vi "总磷总氮通讯.vi"() -> ()   [LabVIEW 2016, in "斯坦道氟化物.lvlib"]
uses:
  <vilib>/Plasmionique/MB Master/MB_Master_Serial/MB_Master_Serial.lvclass
  E:/Program Files (x86)/National Instruments/LabVIEW 2016/vi.lib/Plasmionique/MB Master/MB_Master/MB_Master.lvclass
  <vilib>/Plasmionique/MB Master/MB_Master_TCP/MB_Master_TCP.lvclass
  <vilib>/Utility/config.llb/Write Key (Boolean).vi
  <vilib>/Utility/config.llb/Write Key (String).vi
  <vilib>/Plasmionique/MB Master/MB_Master/MB_Master.lvclass
  <vilib>/Utility/config.llb/NI_LVConfig.lvlib
  <vilib>/Plasmionique/MB Master/MB Master.lvlib
  <vilib>/ptbypt/NI_PtbyPt.lvlib
panel:
  out "启用":bool=TRUE
  out "氨氮状态告警区":u16[](array[numeric])
  out "氨氮测量数据区":u16[](array[numeric])
  out "COD测量数据区":u16[](array[numeric])
  out "COD状态告警区":u16[](array[numeric])
  out "总氮测量数据区":u16[](array[numeric])
  out "总氮状态告警区":u16[](array[numeric])
  out "总磷状态告警区":u16[](array[numeric])
  out "总磷测量数据区":u16[](array[numeric])
  out "状态告警区":T1 {"告警代码" items=["无告警", "缺试剂告警", "缺水样告警", "缺蒸馏水告警", "缺标液告警", "仪表漏液告警", "标定异常告警", "超量程告警", "加热异常", "低试剂预警", "超上限告警", "超下限告警", "仪表内部其他异常", "滴定异常告警", "电极异常告警", "量程切换告警", "参数设置告警", "PH电极电位异常", "电导率电极异常", "浊度光度异常", "溶解氧电极异常", "溶解氧光强异常", "温度异常告警", "PH异常告警", "溶解氧异常告警", "电导率异常告警", "浊度异常告警", "叶绿素异常告警", "藻密度异常告警", "蓝绿藻异常告警", "ORP异常告警", "氨氮异常告警", "清洁刷异常告警", "SD卡异常告警", "蓝牙异常告警", "Wifi异常告警", "流程异常告警"]; "故障代码" items=["无故障", "电机故障", "温度故障", "通讯故障", "滴定故障"]}
  out "测量数据区":T2 {"单位" items=["ug/L", "mg/L", "ppm", "mg/m3", "cm", "ppb", "ug/m3", "%", "nmol/mol", "umol/mol", "MPN/L", "MPN/100ml", "ng/m3", "NTU", "无量纲", "ms/cm", "us/cm", "℃", "mV", "万个/L"]}
  out "status":bool
  out "关键参数区":T3
  in  "读关键参数区":bool
  in  "读状态告警区":bool
  in  "读测量数据区":bool
  in  "站号":u16(ring) items=["总磷"=1, "氨氮"=3]
  in  "停止":bool
  in  "启动":bool
  in  "控制命令":u16(ring) items=["启动测量"=1, "标样核查"=2, "零点核查"=3, "跨度核查"=4, "空白测试"=5, "平行样测试"=6, "加标回收"=7, "空白校准"=8, "标样校准"=9, "初始化（清洗）"=10, "停止测试"=11, "仪器重启"=12, "校时"=13, "模式设置"=14, "测量间隔设置"=15]
  in  "控制命令参数":u16[](array[numeric]) format="%04xH"
  in  "VISA Resource":refnum<visa-resource-name>
  in  "启用模块":bool
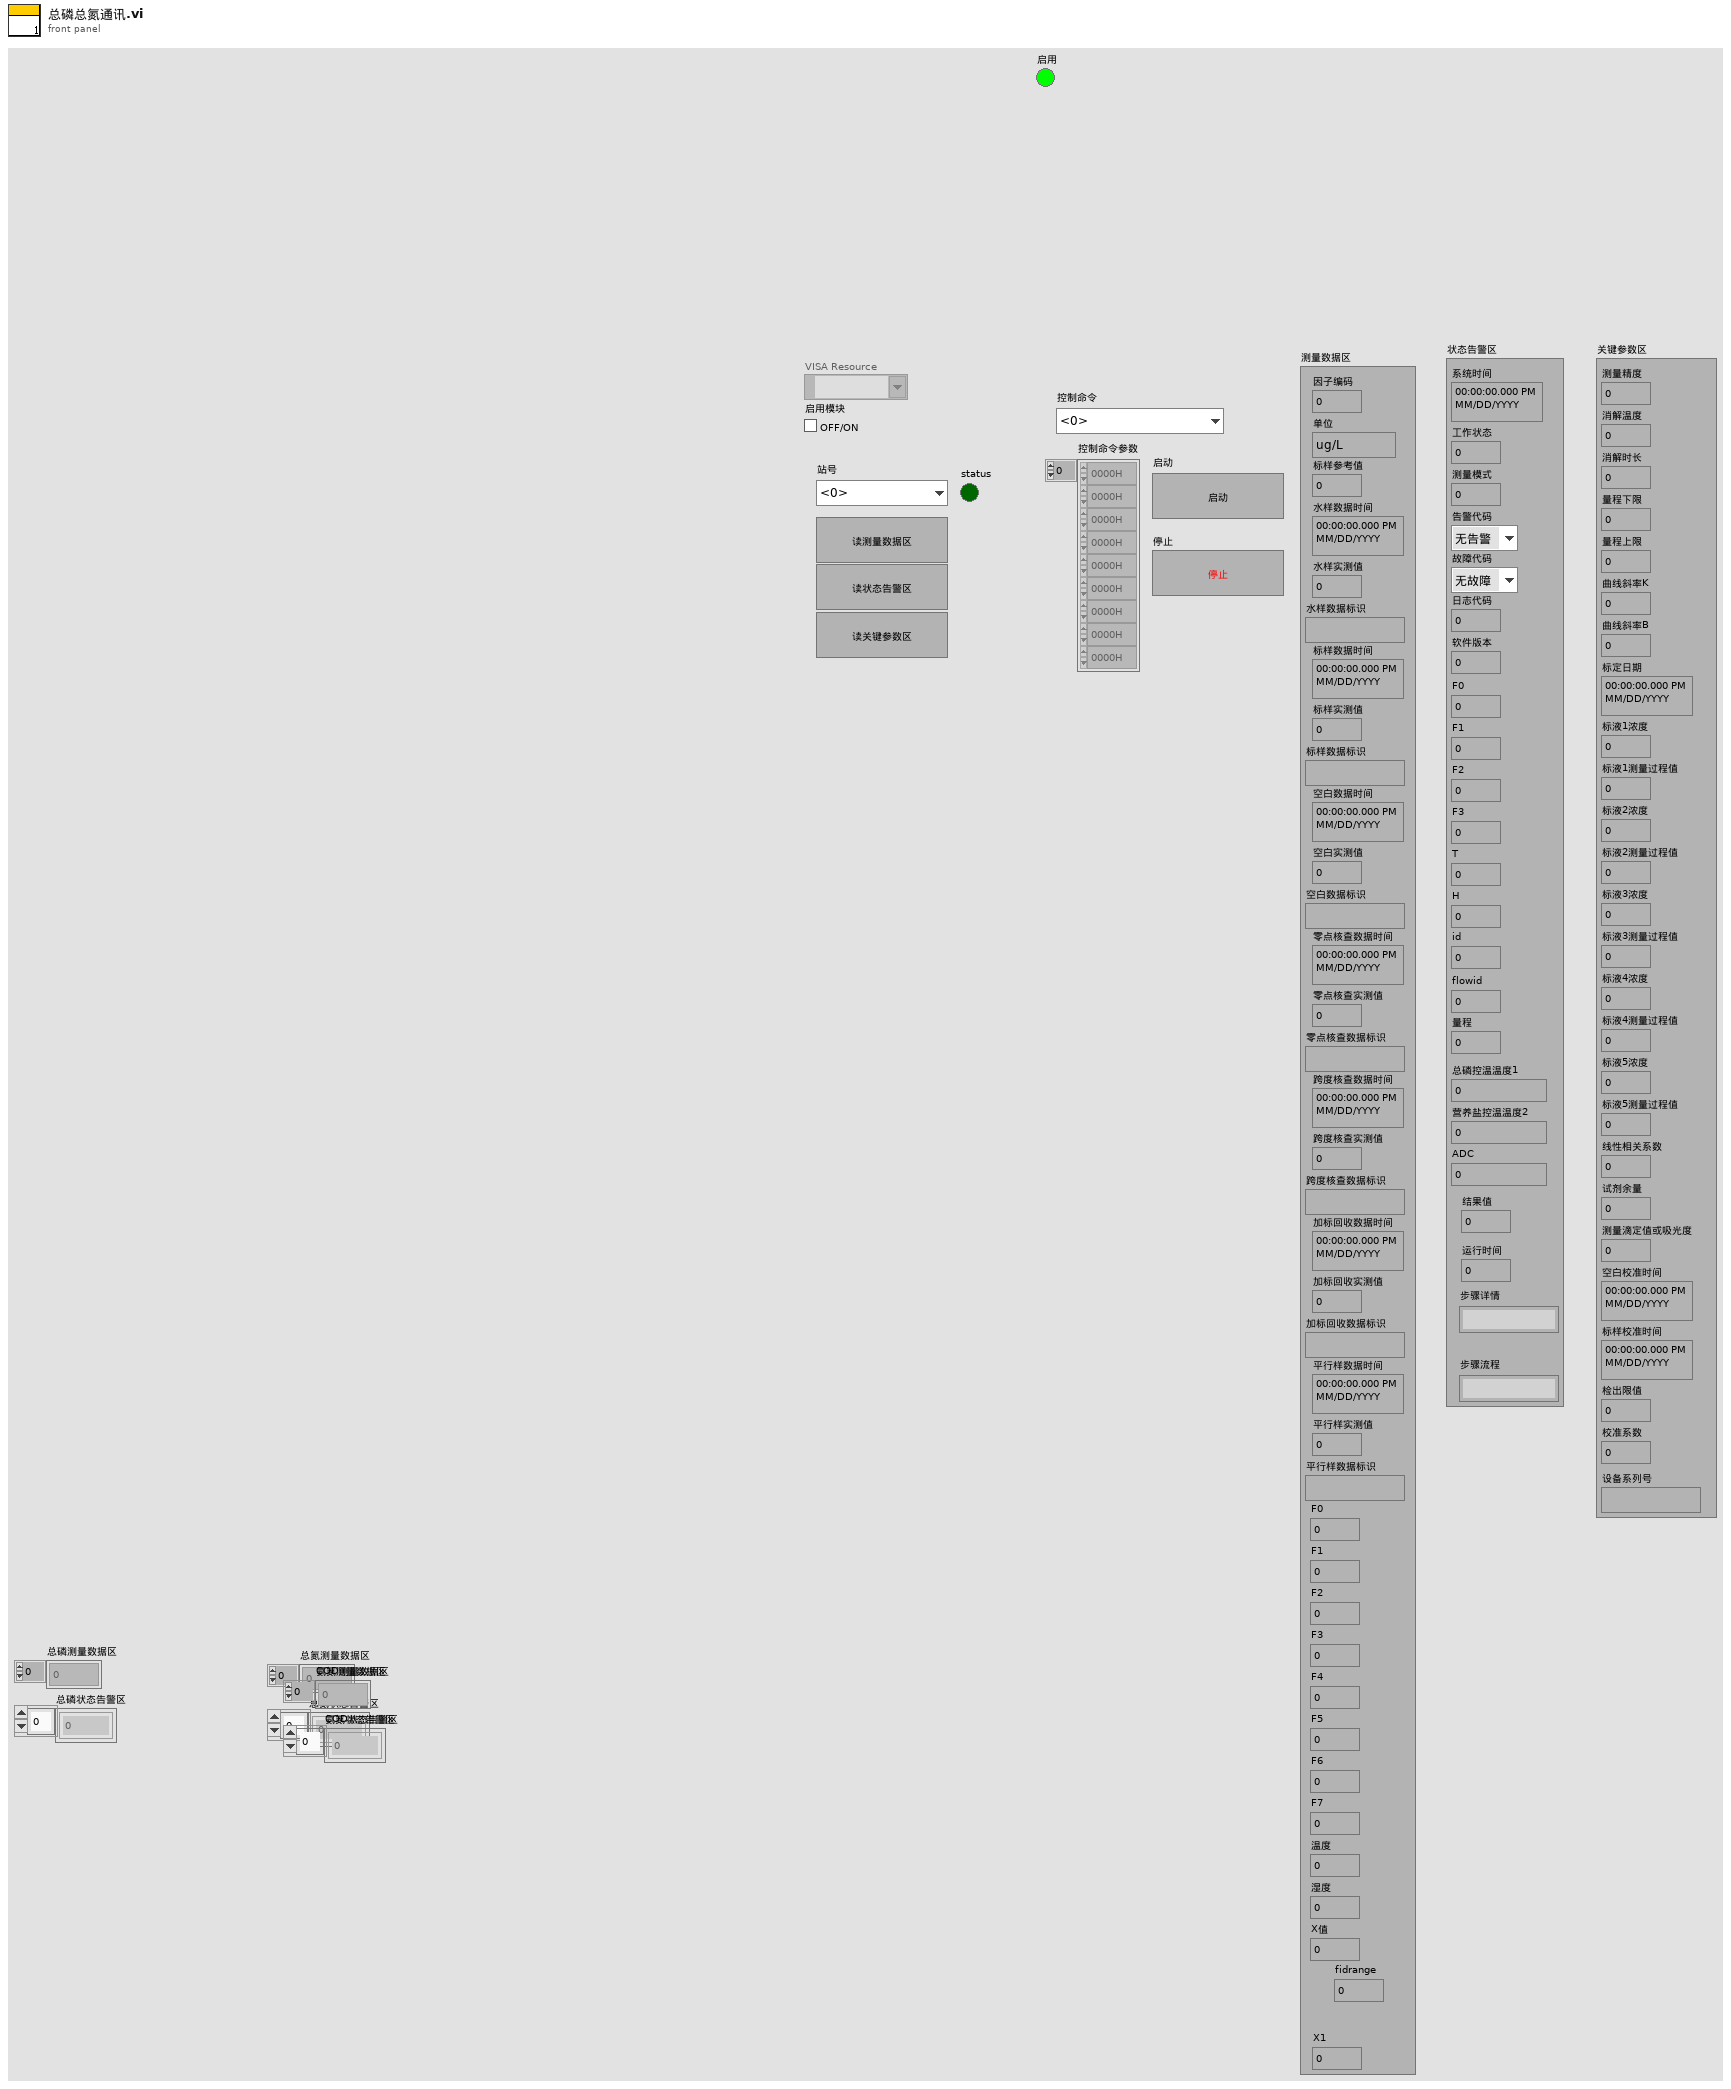
[diagram p1: front panel]
types:
  T1 = cluster{"系统时间":timestamp, "工作状态":u16, "测量模式":u16, "告警代码":u16, "故障代码":u16, "日志代码":u16, "软件版本":u16, "F0":sgl, "F1":sgl, "F2":sgl, "F3":sgl, "T":sgl, "H":sgl, "id":u16, "flowid":u16, "量程":u16, "总磷控温温度1":sgl, "营养盐控温温度2":sgl, "ADC":sgl, "结果值":sgl, "运行时间":u16, "步骤详情":string, "步骤流程":string}
  T2 = cluster{"因子编码":u32, "单位":u16, "标样参考值":sgl, "水样数据时间":timestamp, "水样实测值":sgl, "水样数据标识":string, "标样数据时间":timestamp, "标样实测值":sgl, "标样数据标识":string, "空白数据时间":timestamp, "空白实测值":sgl, "空白数据标识":string, "零点核查数据时间":timestamp, "零点核查实测值":sgl, "零点核查数据标识":string, "跨度核查数据时间":timestamp, "跨度核查实测值":sgl, "跨度核查数据标识":string, "加标回收数据时间":timestamp, "加标回收实测值":sgl, "加标回收数据标识":string, "平行样数据时间":timestamp, "平行样实测值":sgl, "平行样数据标识":string, "F0":sgl, "F1":sgl, "F2":sgl, "F3":sgl, "F4":sgl, "F5":sgl, "F6":sgl, "F7":sgl, "温度":sgl, "湿度":sgl, "X值":sgl, "fidrange":u16, "X1":sgl}
  T3 = cluster{"测量精度":u16, "消解温度":u16, "消解时长":u16, "量程下限":sgl, "量程上限":sgl, "曲线斜率K":sgl, "曲线斜率B":sgl, "标定日期":timestamp, "标液1浓度":sgl, "标液1测量过程值":sgl, "标液2浓度":sgl, "标液2测量过程值":sgl, "标液3浓度":sgl, "标液3测量过程值":sgl, "标液4浓度":sgl, "标液4测量过程值":sgl, "标液5浓度":sgl, "标液5测量过程值":sgl, "线性相关系数":sgl, "试剂余量":u32, "测量滴定值或吸光度":sgl, "空白校准时间":timestamp, "标样校准时间":timestamp, "检出限值":sgl, "校准系数":sgl, "设备系列号":string}
  T4 = cluster{"系统时间":timestamp, "工作状态":u16, "测量模式":enum16{"待机", "连续模式", "周期模式", "定点模式", "受控模式", "手动模式"}, "告警代码":u16, "故障代码":u16, "日志代码":u16, "软件版本":u16, "F0":sgl, "F1":sgl, "F2":sgl, "F3":sgl, "T":sgl, "H":sgl, "id":u16, "flowid":u16, "量程":u16, "总磷控温温度1":sgl, "营养盐控温温度2":sgl, "ADC":sgl}
  T5 = cluster{"因子编码":u32, "单位":u16, "标样参考值":sgl, "水样数据时间":timestamp, "水样实测值":sgl, "水样数据标识":string, "标样数据时间":timestamp, "标样实测值":sgl, "标样数据标识":string, "空白数据时间":timestamp, "空白实测值":sgl, "空白数据标识":string, "零点核查数据时间":timestamp, "零点核查实测值":sgl, "零点核查数据标识":string, "跨度核查数据时间":timestamp, "跨度核查实测值":sgl, "跨度核查数据标识":string, "加标回收数据时间":timestamp, "加标回收实测值":sgl, "加标回收数据标识":string, "平行样数据时间":timestamp, "平行样实测值":sgl, "平行样数据标识":string, "F0":sgl, "F1":sgl, "F2":sgl, "F3":sgl, "F4":sgl, "F5":sgl, "F6":sgl, "F7":sgl, "温度":sgl, "湿度":sgl, "X值":sgl, "fidrange":u16, "X1值":sgl}
  T6 = cluster{"测量精度":u16, "消解温度":u16, "消解时长":u16, "量程下限":sgl, "量程上限":sgl, "曲线斜率K":sgl, "曲线斜率B":sgl, "标定日期":timestamp, "标液1浓度":sgl, "标液1测量过程值":sgl, "标液2浓度":sgl, "标液2测量过程值":sgl, "标液3浓度":sgl, "标液3测量过程值":sgl, "标液4浓度":sgl, "标液4测量过程值":sgl, "标液5浓度":sgl, "标液5测量过程值":sgl, "线性相关系数":sgl, "试剂余量":u32, "测量滴定值或吸光度":sgl, "空白校准时间":timestamp, "标样校准时间":timestamp, "检出限值":sgl, "校准系数":sgl, "设备系列号":string}[]
  T7 = cluster{"系统时间":timestamp, "工作状态":u16, "测量模式":enum16{"待机", "连续模式", "周期模式", "定点模式", "受控模式", "手动模式"}, "告警代码":u16, "故障代码":u16, "日志代码":u16, "软件版本":u16, "F0":sgl, "F1":sgl, "F2":sgl, "F3":sgl, "T":sgl, "H":sgl, "id":u16, "flowid":u16, "量程":u16, "总磷控温温度1":sgl, "营养盐控温温度2":sgl, "ADC":sgl}[]
  T8 = cluster{"因子编码":u32, "单位":u16, "标样参考值":sgl, "水样数据时间":timestamp, "水样实测值":sgl, "水样数据标识":string, "标样数据时间":timestamp, "标样实测值":sgl, "标样数据标识":string, "空白数据时间":timestamp, "空白实测值":sgl, "空白数据标识":string, "零点核查数据时间":timestamp, "零点核查实测值":sgl, "零点核查数据标识":string, "跨度核查数据时间":timestamp, "跨度核查实测值":sgl, "跨度核查数据标识":string, "加标回收数据时间":timestamp, "加标回收实测值":sgl, "加标回收数据标识":string, "平行样数据时间":timestamp, "平行样实测值":sgl, "平行样数据标识":string, "F0":sgl, "F1":sgl, "F2":sgl, "F3":sgl, "F4":sgl, "F5":sgl, "F6":sgl, "F7":sgl, "温度":sgl, "湿度":sgl, "X值":sgl, "fidrange":u16, "X1值":sgl}[]
  T9 = typedef "CODCr交互.ctl" = cluster{"状态告警区":cluster{"系统时间":timestamp, "工作状态":u16, "测量模式":enum16{"待机", "连续模式", "周期模式", "定点模式", "受控模式", "手动模式"}, "告警代码":u16, "故障代码":u16, "日志代码":u16, "软件版本":u16, "F0":sgl, "F1":sgl, "F2":sgl, "F3":sgl, "T":sgl, "H":sgl, "id":u16, "flowid":u16, "量程":u16, "总磷控温温度1":sgl, "营养盐控温温度2":sgl, "ADC":sgl}, "平台试剂余量百分比":sgl, "关键参数":cluster{"测量量程":dbl, "测量精度":dbl, "测量间隔":dbl, "消解温度":dbl, "消解时长":dbl, "空白校准时间":timestamp, "曲线截距":dbl, "曲线斜率":dbl, "测量检出限":dbl, "测量信号值":dbl, "线性相关系数":dbl, "二次多项式系数":dbl, "标样校准时间":timestamp, "稀释倍数":dbl, "三项式系数":dbl, "空白标定系数":dbl, "量程系数":dbl, "F0/ORPA":dbl, "F1/ORPB":dbl, "F2/ORPK":dbl, "F3":dbl, "F4":dbl, "F5":dbl, "F6":dbl, "F7":dbl, "X0/滴定数":dbl, "量程":dbl}, "关键参数改变":bool, "校准信息":cluster{"低标液1浓度":dbl, "低标液1信号值":dbl, "低标液1启用":u16, "低标液2浓度":dbl, "低标液2信号值":dbl, "低标液2启用":u16, "低标液3浓度":dbl, "低标液3信号值":dbl, "低标液3启用":u16, "低标液4浓度":dbl, "低标液4信号值":dbl, "低标液4启用":u16, "低标液5浓度":dbl, "低标液5信号值":dbl, "低标液5启用":u16, "高标液1浓度":dbl, "高标液1信号值":dbl, "高标液1启用":u16, "高标液2浓度":dbl, "高标液2信号值":dbl, "高标液2启用":u16, "高标液3浓度":dbl, "高标液3信号值":dbl, "高标液3启用":u16, "高标液4浓度":dbl, "高标液4信号值":dbl, "高标液4启用":u16, "高标液5浓度":dbl, "高标液5信号值":dbl, "高标液5启用":u16, "低斜率":dbl, "低截距":dbl, "低二次多项式系数":dbl, "低线性相关系数":dbl, "高斜率":dbl, "高截距":dbl, "高二次多项式系数":dbl, "高线性相关系数":dbl}, "校准信息改变":bool, "固件版本号":string}
  T10 = typedef "总磷交互.ctl" = cluster{"状态告警区":cluster{"系统时间":timestamp, "工作状态":u16, "测量模式":enum16{"待机", "连续模式", "周期模式", "定点模式", "受控模式", "手动模式"}, "告警代码":u16, "故障代码":u16, "日志代码":u16, "软件版本":u16, "F0":sgl, "F1":sgl, "F2":sgl, "F3":sgl, "T":sgl, "H":sgl, "id":u16, "flowid":u16, "量程":u16, "总磷控温温度1":sgl, "营养盐控温温度2":sgl, "ADC":sgl}, "平台试剂余量百分比":sgl, "关键参数":cluster{"测量量程":dbl, "测量精度":dbl, "测量间隔":dbl, "消解温度":dbl, "消解时长":dbl, "空白校准时间":timestamp, "曲线截距":dbl, "曲线斜率":dbl, "测量检出限":dbl, "测量信号值":dbl, "线性相关系数":dbl, "二次多项式系数":dbl, "标样校准时间":timestamp, "稀释倍数":dbl, "三项式系数":dbl, "空白标定系数":dbl, "量程系数":dbl, "F0/ORPA":dbl, "F1/ORPB":dbl, "F2/ORPK":dbl, "F3":dbl, "F4":dbl, "F5":dbl, "F6":dbl, "F7":dbl, "X0/滴定数":dbl, "量程":dbl}, "关键参数改变":bool, "校准信息":cluster{"低标液1浓度":dbl, "低标液1信号值":dbl, "低标液1启用":u16, "低标液2浓度":dbl, "低标液2信号值":dbl, "低标液2启用":u16, "低标液3浓度":dbl, "低标液3信号值":dbl, "低标液3启用":u16, "低标液4浓度":dbl, "低标液4信号值":dbl, "低标液4启用":u16, "低标液5浓度":dbl, "低标液5信号值":dbl, "低标液5启用":u16, "高标液1浓度":dbl, "高标液1信号值":dbl, "高标液1启用":u16, "高标液2浓度":dbl, "高标液2信号值":dbl, "高标液2启用":u16, "高标液3浓度":dbl, "高标液3信号值":dbl, "高标液3启用":u16, "高标液4浓度":dbl, "高标液4信号值":dbl, "高标液4启用":u16, "高标液5浓度":dbl, "高标液5信号值":dbl, "高标液5启用":u16, "低斜率":dbl, "低截距":dbl, "低二次多项式系数":dbl, "低线性相关系数":dbl, "高斜率":dbl, "高截距":dbl, "高二次多项式系数":dbl, "高线性相关系数":dbl}, "校准信息改变":bool, "固件版本号":string}
  T11 = typedef "总氮交互.ctl" = cluster{"状态告警区":cluster{"系统时间":timestamp, "工作状态":u16, "测量模式":enum16{"待机", "连续模式", "周期模式", "定点模式", "受控模式", "手动模式"}, "告警代码":u16, "故障代码":u16, "日志代码":u16, "软件版本":u16, "F0":sgl, "F1":sgl, "F2":sgl, "F3":sgl, "T":sgl, "H":sgl, "id":u16, "flowid":u16, "量程":u16, "总磷控温温度1":sgl, "营养盐控温温度2":sgl, "ADC":sgl}, "平台试剂余量百分比":sgl, "关键参数":cluster{"测量量程":dbl, "测量精度":dbl, "测量间隔":dbl, "消解温度":dbl, "消解时长":dbl, "空白校准时间":timestamp, "曲线截距":dbl, "曲线斜率":dbl, "测量检出限":dbl, "测量信号值":dbl, "线性相关系数":dbl, "二次多项式系数":dbl, "标样校准时间":timestamp, "稀释倍数":dbl, "三项式系数":dbl, "空白标定系数":dbl, "量程系数":dbl, "F0/ORPA":dbl, "F1/ORPB":dbl, "F2/ORPK":dbl, "F3":dbl, "F4":dbl, "F5":dbl, "F6":dbl, "F7":dbl, "X0/滴定数":dbl, "量程":dbl}, "关键参数改变":bool, "校准信息":cluster{"低标液1浓度":dbl, "低标液1信号值":dbl, "低标液1启用":u16, "低标液2浓度":dbl, "低标液2信号值":dbl, "低标液2启用":u16, "低标液3浓度":dbl, "低标液3信号值":dbl, "低标液3启用":u16, "低标液4浓度":dbl, "低标液4信号值":dbl, "低标液4启用":u16, "低标液5浓度":dbl, "低标液5信号值":dbl, "低标液5启用":u16, "高标液1浓度":dbl, "高标液1信号值":dbl, "高标液1启用":u16, "高标液2浓度":dbl, "高标液2信号值":dbl, "高标液2启用":u16, "高标液3浓度":dbl, "高标液3信号值":dbl, "高标液3启用":u16, "高标液4浓度":dbl, "高标液4信号值":dbl, "高标液4启用":u16, "高标液5浓度":dbl, "高标液5信号值":dbl, "高标液5启用":u16, "低斜率":dbl, "低截距":dbl, "低二次多项式系数":dbl, "低线性相关系数":dbl, "高斜率":dbl, "高截距":dbl, "高二次多项式系数":dbl, "高线性相关系数":dbl}, "校准信息改变":bool, "固件版本号":string}
  T12 = typedef "氨氮交互.ctl" = cluster{"状态告警区":cluster{"系统时间":timestamp, "工作状态":u16, "测量模式":enum16{"待机", "连续模式", "周期模式", "定点模式", "受控模式", "手动模式"}, "告警代码":u16, "故障代码":u16, "日志代码":u16, "软件版本":u16, "F0":sgl, "F1":sgl, "F2":sgl, "F3":sgl, "T":sgl, "H":sgl, "id":u16, "flowid":u16, "量程":u16, "总磷控温温度1":sgl, "营养盐控温温度2":sgl, "ADC":sgl}, "平台试剂余量百分比":sgl, "关键参数":cluster{"测量量程":dbl, "测量精度":dbl, "测量间隔":dbl, "消解温度":dbl, "消解时长":dbl, "空白校准时间":timestamp, "曲线截距":dbl, "曲线斜率":dbl, "测量检出限":dbl, "测量信号值":dbl, "线性相关系数":dbl, "二次多项式系数":dbl, "标样校准时间":timestamp, "稀释倍数":dbl, "三项式系数":dbl, "空白标定系数":dbl, "量程系数":dbl, "F0/ORPA":dbl, "F1/ORPB":dbl, "F2/ORPK":dbl, "F3":dbl, "F4":dbl, "F5":dbl, "F6":dbl, "F7":dbl, "X0/滴定数":dbl, "量程":dbl}, "关键参数改变":bool, "校准信息":cluster{"低标液1浓度":dbl, "低标液1信号值":dbl, "低标液1启用":u16, "低标液2浓度":dbl, "低标液2信号值":dbl, "低标液2启用":u16, "低标液3浓度":dbl, "低标液3信号值":dbl, "低标液3启用":u16, "低标液4浓度":dbl, "低标液4信号值":dbl, "低标液4启用":u16, "低标液5浓度":dbl, "低标液5信号值":dbl, "低标液5启用":u16, "高标液1浓度":dbl, "高标液1信号值":dbl, "高标液1启用":u16, "高标液2浓度":dbl, "高标液2信号值":dbl, "高标液2启用":u16, "高标液3浓度":dbl, "高标液3信号值":dbl, "高标液3启用":u16, "高标液4浓度":dbl, "高标液4信号值":dbl, "高标液4启用":u16, "高标液5浓度":dbl, "高标液5信号值":dbl, "高标液5启用":u16, "低斜率":dbl, "低截距":dbl, "低二次多项式系数":dbl, "低线性相关系数":dbl, "高斜率":dbl, "高截距":dbl, "高二次多项式系数":dbl, "高线性相关系数":dbl}, "校准信息改变":bool, "固件版本号":string}
  T13 = typedef "操作日志字段定义.ctl" = cluster{"时间":timestamp, "参数":string, "日志信息":string, "流程参数":string}
  T14 = typedef "NI_LVConfig.lvlib/Config Data RefNum.ctl" = refnum<k1>
  T15 = enum8{"Enabled", "Disabled", "Disabled and Grayed Out"}
  T16 = cluster{"baud rate (bps)":u32, "stop bits":u16, "parity":u16, "flow control":u16, "timeout":u32, "retries":i32}
  T17 = typedef "工况数据.ctl" = cluster{"time":string, "data":cluster{"ups":cluster{"ups":cluster{"input_voltage":ext, "input_frequency":ext, "output_voltage":ext, "output_current":ext, "output_frequency":ext, "output_active_power":ext, "output_apparent_power":ext, "load_rate":ext, "cabinet_temperature":ext, "battery_voltage":ext, "remaining_battery_capacity":ext, "power_on_status":string, "power_supply_mode":string, "fault":bool, "battery_low_voltage":bool, "mains_supply_abnormality":bool}, "启用":bool}, "air_conditioner":cluster{"air_conditioner":cluster{"cabinet_temperature":ext, "air_supply_temperature":ext, "voltage":ext, "current":ext, "compressor_status":string, "Internal_fan_status":string, "external_fan_status":string, "heating_state":string, "refrigeration_state":bool, "high_temperature_alarm":bool, "low_temperature_alarm":bool, "heater_fault":bool, "temperature_sensor_fault":bool, "high_voltage_alarm":bool, "low_voltage_alarm":bool, "refrigeration_start_point":ext, "refrigeration_sensitive_point":ext, "heating_start_point":ext, "heating_sensitive_point":ext, "high_temperature_alarm_point":ext, "low_temperature_alarm_point":ext}, "启用":bool}, "smoke_sensor":cluster{"smoke_sensor":cluster{"trigger_alarm":bool}, "启用":bool}, "water_immersion_sensor":cluster{"water_immersion_sensor":cluster{"trigger_alarm":bool}, "启用":bool}, "temperature_and_humidity_sensor":cluster{"temperature_and_humidity_sensor":cluster{"current_temperature":ext, "current_humidity":ext, "room_temperature_alarm":bool, "humidity_alarm":bool}, "启用":bool}, "gps":cluster{"gps":cluster{"current_longitude":ext, "current_latitude":ext, "launch_longitude":ext, "launch_latitude":ext, "shift_alarm":bool}, "启用":bool}, "solar_controller":cluster{"solar_controller":cluster{"array_voltage":ext, "array_current":ext, "generating_power":ext, "battery_voltage":dbl, "battery_current":ext, "ceiling_voltage":ext, "minimum_voltage":ext, "battery_temperature":ext, "remaining_battery_capacity":ext, "load_voltage":ext, "load_current":ext, "load_power":ext, "equipment_temperature":ext, "accumulated_electricity_consumption_of_the_day":ext, "accumulated_electricity_consumption_of_the_current_month":ext, "accumulated_electricity_consumption_in_the_current_year":ext, "total_accumulated_power_consumption":ext, "accumulated_charging_capacity_of_the_day":ext, "accumulated_charging_amount_of_the_current_month":ext, "accumulated_charging_capacity_of_the_current_year":ext, "total_cumulative_charge":ext}, "启用":bool}, "solar_controller_2":cluster{"solar_controller_2":cluster{"array_voltage":ext, "array_current":ext, "generating_power":ext, "battery_voltage":dbl, "battery_current":ext, "ceiling_voltage":ext, "minimum_voltage":ext, "battery_temperature":ext, "remaining_battery_capacity":ext, "load_voltage":ext, "load_current":ext, "load_power":ext, "equipment_temperature":ext, "accumulated_electricity_consumption_of_the_day":ext, "accumulated_electricity_consumption_of_the_current_month":ext, "accumulated_electricity_consumption_in_the_current_year":ext, "total_accumulated_power_consumption":ext, "accumulated_charging_capacity_of_the_day":ext, "accumulated_charging_amount_of_the_current_month":ext, "accumulated_charging_capacity_of_the_current_year":ext, "total_cumulative_charge":ext}, "启用":bool}, "NH3":cluster{"NH3":cluster{"F0":ext, "F1":ext, "syringe_temperature":ext, "alarm_step":dbl, "X0":ext}, "启用":bool}, "TP":cluster{"TP":cluster{"F0":ext, "F1":ext, "F2":ext, "F3":ext, "digestion_temperature":ext, "constant_temperature":ext, "syringe_temperature":ext, "alarm_step":dbl, "X0":ext}, "启用":bool}, "TN":cluster{"TN":cluster{"F0":ext, "F1":ext, "F2":ext, "F3":ext, "F4":ext, "F5":ext, "F6":ext, "F7":ext, "digestion_temperature":ext, "constant_temperature":ext, "syringe_temperature":ext, "alarm_step":dbl, "X0":ext}, "启用":bool}, "CODMn":cluster{"CODMn":cluster{"temperature_curve":ext[], "titration_curve":ext[], "F0":ext, "F1":ext, "F2":ext, "F3":ext, "F4":ext, "F5":ext, "A":ext, "B":ext, "K":ext}, "启用":bool}, "CODCr":cluster{"CODCr":cluster{"temperature_curve":ext[], "F0":ext, "F1":ext, "reagent_sensor":ext}, "启用":bool}}}
  T18 = cluster{"系统时间":timestamp, "工作状态":u16, "测量模式":enum16{"待机", "连续模式", "周期模式", "定点模式", "受控模式", "手动模式"}, "告警代码":u16, "故障代码":u16, "日志代码":u16, "软件版本":u16, "F0":sgl, "F1":sgl, "F2":sgl, "F3":sgl, "T":sgl, "H":sgl, "id":u16, "flowid":u16, "量程":u16, "总磷控温温度1":sgl, "营养盐控温温度2":sgl, "ADC":sgl, "结果值":sgl, "运行时间":u16, "步骤详情":string, "步骤流程":string}
  T19 = typedef "斯坦道氟化物.lvlib/关键参数.ctl" = cluster{"测量量程":sgl, "测量检出限":sgl, "测量精度":sgl, "测量间隔":sgl, "消解温度":sgl, "消解时长":sgl, "三项式系数":sgl, "二次多项式系数":sgl, "曲线斜率":sgl, "曲线截距":sgl, "线性相关系数":sgl, "空白校准时间":timestamp, "标样校准时间":timestamp, "测量信号值":sgl, "稀释倍数":sgl, "空白标定系数":sgl, "量程系数":sgl}
  T20 = cluster{"测量量程":dbl, "测量精度":dbl, "测量间隔":dbl, "消解温度":dbl, "消解时长":dbl, "空白校准时间":timestamp, "曲线截距":dbl, "曲线斜率":dbl, "测量检出限":dbl, "测量信号值":dbl, "线性相关系数":dbl, "二次多项式系数":dbl, "标样校准时间":timestamp, "稀释倍数":dbl, "三项式系数":dbl, "空白标定系数":dbl, "量程系数":dbl, "F0/ORPA":dbl, "F1/ORPB":dbl, "F2/ORPK":dbl, "F3":dbl, "F4":dbl, "F5":dbl, "F6":dbl, "F7":dbl, "X0/滴定数":dbl, "量程":dbl}
  T21 = cluster{"低标液1浓度":dbl, "低标液1信号值":dbl, "低标液1启用":u16, "低标液2浓度":dbl, "低标液2信号值":dbl, "低标液2启用":u16, "低标液3浓度":dbl, "低标液3信号值":dbl, "低标液3启用":u16, "低标液4浓度":dbl, "低标液4信号值":dbl, "低标液4启用":u16, "低标液5浓度":dbl, "低标液5信号值":dbl, "低标液5启用":u16, "高标液1浓度":dbl, "高标液1信号值":dbl, "高标液1启用":u16, "高标液2浓度":dbl, "高标液2信号值":dbl, "高标液2启用":u16, "高标液3浓度":dbl, "高标液3信号值":dbl, "高标液3启用":u16, "高标液4浓度":dbl, "高标液4信号值":dbl, "高标液4启用":u16, "高标液5浓度":dbl, "高标液5信号值":dbl, "高标液5启用":u16, "低斜率":dbl, "低截距":dbl, "低二次多项式系数":dbl, "低线性相关系数":dbl, "高斜率":dbl, "高截距":dbl, "高二次多项式系数":dbl, "高线性相关系数":dbl}
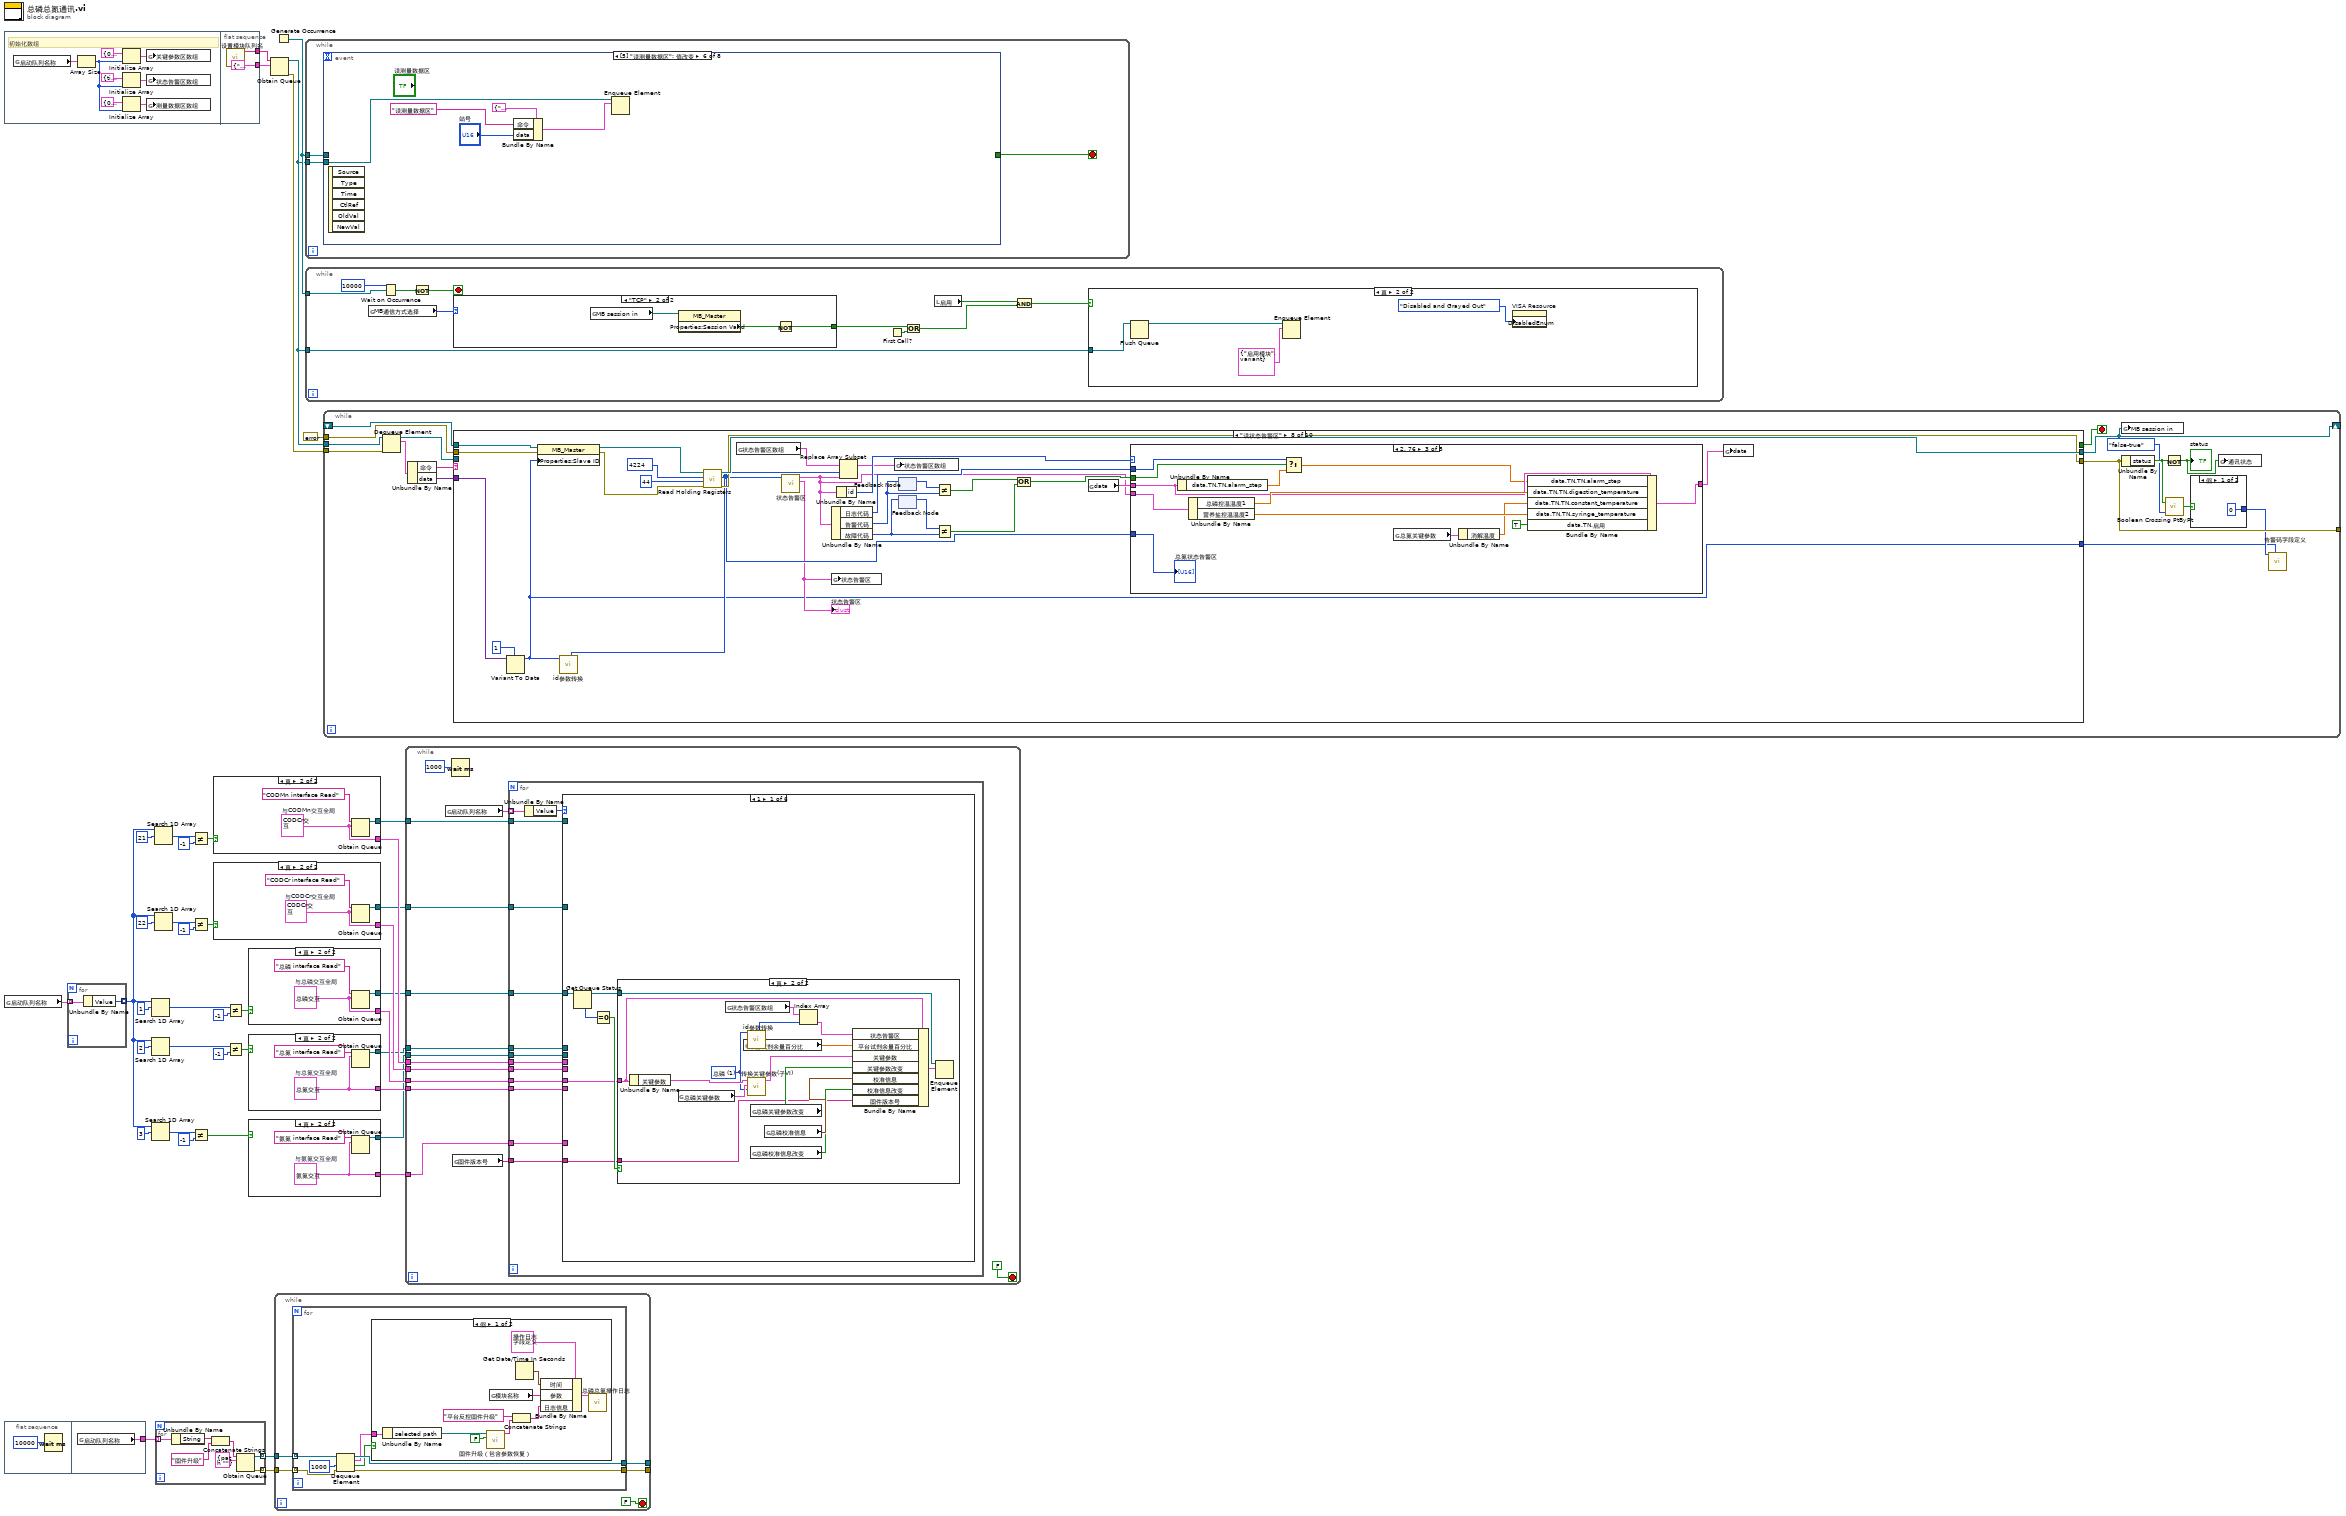
[diagram p0: block diagram]
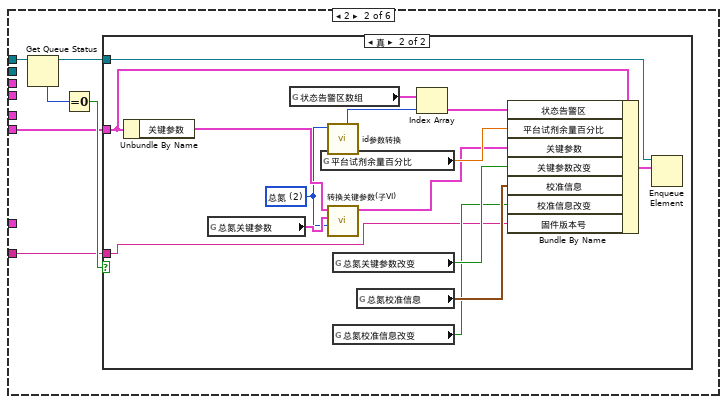
[diagram p9: hidden frame]
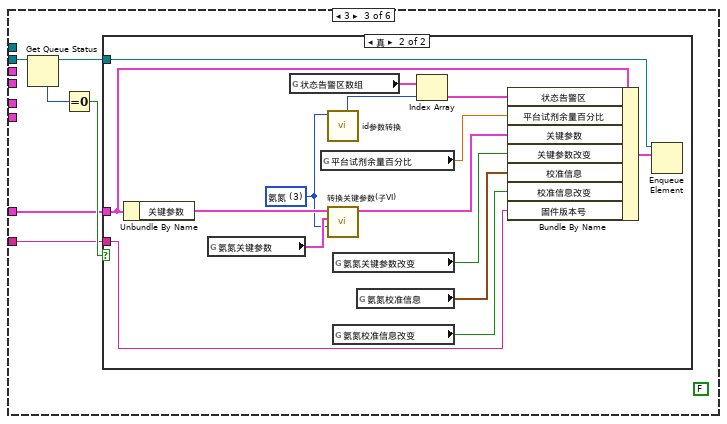
[diagram p11: hidden frame]
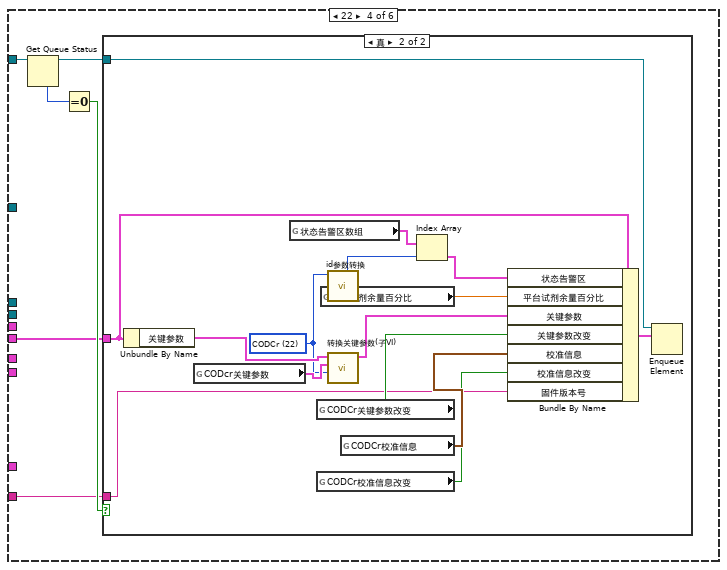
[diagram p13: hidden frame]
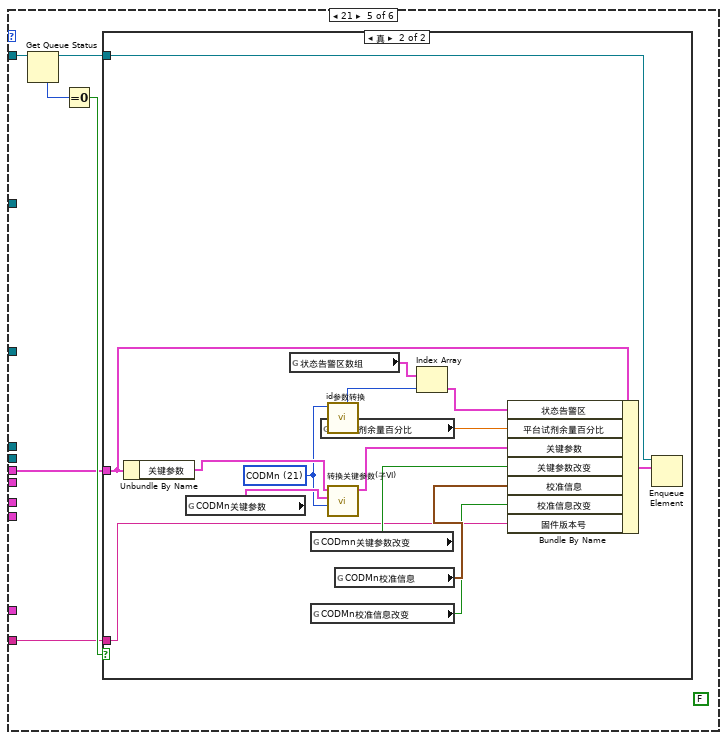
[diagram p15: hidden frame]
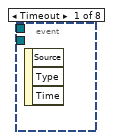
[diagram p20: hidden frame]
diagram:
  n1 = flat-sequence {
    tunnel: [cluster{"命令":string, "data":variant} {"命令"="", "data"=variant}] -> w41
    tunnel: [w50] -> w36
    frame #0 {
      # "初始化数组"
      n2 = global read "model config var.vi" "启动队列名称"() -> (w43:cluster{"String":string, "Value":u16}[])
      n3 = Array Size(array=w43) -> (size(s)=w42:i32)
      n4 = Initialize Array(T3 {"测量精度"=0, "消解温度"=0, "消解时长"=0, "量程下限"=0.0, "量程上限"=0.0, "曲线斜率K"=0.0, "曲线斜率B"=0.0, "标定日期"=timestamp(0 s since 1904-01-01), "标液1浓度"=0.0, "标液1测量过程值"=0.0, "标液2浓度"=0.0, "标液2测量过程值"=0.0, "标液3浓度"=0.0, "标液3测量过程值"=0.0, "标液4浓度"=0.0, "标液4测量过程值"=0.0, "标液5浓度"=0.0, "标液5测量过程值"=0.0, "线性相关系数"=0.0, "试剂余量"=0, "测量滴定值或吸光度"=0.0, "空白校准时间"=timestamp(0 s since 1904-01-01), "标样校准时间"=timestamp(0 s since 1904-01-01), "检出限值"=0.0, "校准系数"=0.0, "设备系列号"=""} ("关键参数区"), w42) -> (w47:T6)
      n5 = Initialize Array(T4 {"系统时间"=timestamp(0 s since 1904-01-01), "工作状态"=0, "测量模式"=enum."待机", "告警代码"=0, "故障代码"=0, "日志代码"=0, "软件版本"=0, "F0"=0.0, "F1"=0.0, "F2"=0.0, "F3"=0.0, "T"=0.0, "H"=0.0, "id"=0, "flowid"=0, "量程"=0, "总磷控温温度1"=0.0, "营养盐控温温度2"=0.0, "ADC"=0.0} ("状态告警区"), w42) -> (w46:T7)
      n6 = Initialize Array(T5 {"因子编码"=0, "单位"=0, "标样参考值"=0.0, "水样数据时间"=timestamp(0 s since 1904-01-01), "水样实测值"=0.0, "水样数据标识"="", "标样数据时间"=timestamp(0 s since 1904-01-01), "标样实测值"=0.0, "标样数据标识"="", "空白数据时间"=timestamp(0 s since 1904-01-01), "空白实测值"=0.0, "空白数据标识"="", "零点核查数据时间"=timestamp(0 s since 1904-01-01), "零点核查实测值"=0.0, "零点核查数据标识"="", "跨度核查数据时间"=timestamp(0 s since 1904-01-01), "跨度核查实测值"=0.0, "跨度核查数据标识"="", "加标回收数据时间"=timestamp(0 s since 1904-01-01), "加标回收实测值"=0.0, "加标回收数据标识"="", "平行样数据时间"=timestamp(0 s since 1904-01-01), "平行样实测值"=0.0, "平行样数据标识"="", "F0"=0.0, "F1"=0.0, "F2"=0.0, "F3"=0.0, "F4"=0.0, "F5"=0.0, "F6"=0.0, "F7"=0.0, "温度"=0.0, "湿度"=0.0, "X值"=0.0, "fidrange"=0, "X1值"=0.0} ("测量数据区"), w42) -> (w49:T8)
      n7 = global write "VAR总磷总氮全局变量.vi" "关键参数区数组"(w47) -> ()
      n8 = global write "VAR总磷总氮全局变量.vi" "状态告警区数组"(w46) -> ()
      n9 = global write "VAR总磷总氮全局变量.vi" "测量数据区数组"(w49) -> ()
    }
    frame #1 {
      n10 = call "设置模块队列名.vi"() -> ("Msg"=w50:string)  [unwired: 5 in]
    }
  }
  n11 = global read "model config var.vi" "启动队列名称"() -> (w25:cluster{"String":string, "Value":u16}[])
  n12 = flat-sequence {
    tunnel: [w53] -> w3
    frame #0 {
      n13 = Wait (ms)(milliseconds to wait=u32 10000 ("等待时间（毫秒）")) -> ()  [unwired: 1 out]
    }
    frame #1 {
      n14 = global read "model config var.vi" "启动队列名称"() -> (w53:cluster{"String":string, "Value":u16}[])
    }
  }
  n15 = for {
    tunnel: w25 -> [w55] mode=indexing
    tunnel: [w54] -> w5 mode=indexing
    n16 = Unbundle By Name(w55) -> ("Value"=w54:u16)
  }
  n17 = Search 1D Array(1D array=w5, element=u16 1 ("元素")) -> (index of element=w15:i32)  [unwired: 1 in]
  n18 = Search 1D Array(1D array=w5, element=u16 2 ("元素")) -> (index of element=w11:i32)  [unwired: 1 in]
  n19 = Search 1D Array(1D array=w5, element=u16 3 ("元素")) -> (index of element=w7:i32)  [unwired: 1 in]
  n20 = Search 1D Array(1D array=w5, element=u16 21 ("元素")) -> (index of element=w23:i32)  [unwired: 1 in]
  n21 = Search 1D Array(1D array=w5, element=u16 22 ("元素")) -> (index of element=w19:i32)  [unwired: 1 in]
  n22 = for {
    tunnel: w3 -> [w62] mode=indexing
    tunnel: [w57] -> w2 mode=indexing
    tunnel: [w56] -> w1 mode=indexing
    n23 = Unbundle By Name(w62) -> ("String"=w58:string)
    n24 = Concatenate Strings(w58, "固件升级" ("字符串")) -> (w60:string)
    n25 = Obtain Queue(name (unnamed)=w60, element data type=cluster{"selected path":path} {"selected path"=path ""}) -> (queue out=w57:refnum<queue>, error out=w56:errorcluster)  [unwired: 3 in, 1 out]
  }
  n26 = Not Equal?(x=w23, y=-1) -> (x != y?=w21:bool)
  n27 = Not Equal?(x=w19, y=-1) -> (x != y?=w17:bool)
  n28 = Not Equal?(x=w7, y=-1) -> (x != y?=w4:bool)
  n29 = case shown="真" w21 {
    tunnel: [_ w64] -> w35
    tunnel: [_ w63] -> w34
    frame False {
    }
    frame True {
      w63 = T9 {"状态告警区"={"系统时间"=timestamp(0 s since 1904-01-01), "工作状态"=0, "测量模式"=enum."待机", "告警代码"=0, "故障代码"=0, "日志代码"=0, "软件版本"=0, "F0"=0.0, "F1"=0.0, "F2"=0.0, "F3"=0.0, "T"=0.0, "H"=0.0, "id"=0, "flowid"=0, "量程"=0, "总磷控温温度1"=0.0, "营养盐控温温度2"=0.0, "ADC"=0.0}, "平台试剂余量百分比"=0.0, "关键参数"={"测量量程"=0.0, "测量精度"=0.0, "测量间隔"=0.0, "消解温度"=0.0, "消解时长"=0.0, "空白校准时间"=timestamp(0 s since 1904-01-01), "曲线截距"=0.0, "曲线斜率"=0.0, "测量检出限"=0.0, "测量信号值"=0.0, "线性相关系数"=0.0, "二次多项式系数"=0.0, "标样校准时间"=timestamp(0 s since 1904-01-01), "稀释倍数"=0.0, "三项式系数"=0.0, "空白标定系数"=0.0, "量程系数"=0.0, "F0/ORPA"=0.0, "F1/ORPB"=0.0, "F2/ORPK"=0.0, "F3"=0.0, "F4"=0.0, "F5"=0.0, "F6"=0.0, "F7"=0.0, "X0/滴定数"=0.0, "量程"=0.0}, "关键参数改变"=FALSE, "校准信息"={"低标液1浓度"=0.0, "低标液1信号值"=0.0, "低标液1启用"=0, "低标液2浓度"=0.0, "低标液2信号值"=0.0, "低标液2启用"=0, "低标液3浓度"=0.0, "低标液3信号值"=0.0, "低标液3启用"=0, "低标液4浓度"=0.0, "低标液4信号值"=0.0, "低标液4启用"=0, "低标液5浓度"=0.0, "低标液5信号值"=0.0, "低标液5启用"=0, "高标液1浓度"=0.0, "高标液1信号值"=0.0, "高标液1启用"=0, "高标液2浓度"=0.0, "高标液2信号值"=0.0, "高标液2启用"=0, "高标液3浓度"=0.0, "高标液3信号值"=0.0, "高标液3启用"=0, "高标液4浓度"=0.0, "高标液4信号值"=0.0, "高标液4启用"=0, "高标液5浓度"=0.0, "高标液5信号值"=0.0, "高标液5启用"=0, "低斜率"=0.0, "低截距"=0.0, "低二次多项式系数"=0.0, "低线性相关系数"=0.0, "高斜率"=0.0, "高截距"=0.0, "高二次多项式系数"=0.0, "高线性相关系数"=0.0}, "校准信息改变"=FALSE, "固件版本号"=""}  # 与CODMn交互全局
      n30 = Obtain Queue(name (unnamed)="CODMn interface Read" ("写入方名称"), element data type=w63) -> (queue out=w64:refnum<queue>)  [unwired: 3 in, 2 out]
    }
  }
  n31 = case shown="真" w17 {
    tunnel: [_ w67] -> w33
    tunnel: [_ w66] -> w32
    frame False {
    }
    frame True {
      w66 = T9 {"状态告警区"={"系统时间"=timestamp(0 s since 1904-01-01), "工作状态"=0, "测量模式"=enum."待机", "告警代码"=0, "故障代码"=0, "日志代码"=0, "软件版本"=0, "F0"=0.0, "F1"=0.0, "F2"=0.0, "F3"=0.0, "T"=0.0, "H"=0.0, "id"=0, "flowid"=0, "量程"=0, "总磷控温温度1"=0.0, "营养盐控温温度2"=0.0, "ADC"=0.0}, "平台试剂余量百分比"=0.0, "关键参数"={"测量量程"=0.0, "测量精度"=0.0, "测量间隔"=0.0, "消解温度"=0.0, "消解时长"=0.0, "空白校准时间"=timestamp(0 s since 1904-01-01), "曲线截距"=0.0, "曲线斜率"=0.0, "测量检出限"=0.0, "测量信号值"=0.0, "线性相关系数"=0.0, "二次多项式系数"=0.0, "标样校准时间"=timestamp(0 s since 1904-01-01), "稀释倍数"=0.0, "三项式系数"=0.0, "空白标定系数"=0.0, "量程系数"=0.0, "F0/ORPA"=0.0, "F1/ORPB"=0.0, "F2/ORPK"=0.0, "F3"=0.0, "F4"=0.0, "F5"=0.0, "F6"=0.0, "F7"=0.0, "X0/滴定数"=0.0, "量程"=0.0}, "关键参数改变"=FALSE, "校准信息"={"低标液1浓度"=0.0, "低标液1信号值"=0.0, "低标液1启用"=0, "低标液2浓度"=0.0, "低标液2信号值"=0.0, "低标液2启用"=0, "低标液3浓度"=0.0, "低标液3信号值"=0.0, "低标液3启用"=0, "低标液4浓度"=0.0, "低标液4信号值"=0.0, "低标液4启用"=0, "低标液5浓度"=0.0, "低标液5信号值"=0.0, "低标液5启用"=0, "高标液1浓度"=0.0, "高标液1信号值"=0.0, "高标液1启用"=0, "高标液2浓度"=0.0, "高标液2信号值"=0.0, "高标液2启用"=0, "高标液3浓度"=0.0, "高标液3信号值"=0.0, "高标液3启用"=0, "高标液4浓度"=0.0, "高标液4信号值"=0.0, "高标液4启用"=0, "高标液5浓度"=0.0, "高标液5信号值"=0.0, "高标液5启用"=0, "低斜率"=0.0, "低截距"=0.0, "低二次多项式系数"=0.0, "低线性相关系数"=0.0, "高斜率"=0.0, "高截距"=0.0, "高二次多项式系数"=0.0, "高线性相关系数"=0.0}, "校准信息改变"=FALSE, "固件版本号"=""}  # 与CODCr交互全局
      n32 = Obtain Queue(name (unnamed)="CODCr interface Read" ("写入方名称"), element data type=w66) -> (queue out=w67:refnum<queue>)  [unwired: 3 in, 2 out]
    }
  }
  n33 = Not Equal?(x=w15, y=-1) -> (x != y?=w13:bool)
  n34 = Not Equal?(x=w11, y=-1) -> (x != y?=w9:bool)
  n35 = case shown="真" w13 {
    tunnel: [_ w70] -> w31
    tunnel: [_ w69] -> w30
    frame False {
    }
    frame True {
      w69 = T10 {"状态告警区"={"系统时间"=timestamp(0 s since 1904-01-01), "工作状态"=0, "测量模式"=enum."待机", "告警代码"=0, "故障代码"=0, "日志代码"=0, "软件版本"=0, "F0"=0.0, "F1"=0.0, "F2"=0.0, "F3"=0.0, "T"=0.0, "H"=0.0, "id"=0, "flowid"=0, "量程"=0, "总磷控温温度1"=0.0, "营养盐控温温度2"=0.0, "ADC"=0.0}, "平台试剂余量百分比"=0.0, "关键参数"={"测量量程"=0.0, "测量精度"=0.0, "测量间隔"=0.0, "消解温度"=0.0, "消解时长"=0.0, "空白校准时间"=timestamp(0 s since 1904-01-01), "曲线截距"=0.0, "曲线斜率"=0.0, "测量检出限"=0.0, "测量信号值"=0.0, "线性相关系数"=0.0, "二次多项式系数"=0.0, "标样校准时间"=timestamp(0 s since 1904-01-01), "稀释倍数"=0.0, "三项式系数"=0.0, "空白标定系数"=0.0, "量程系数"=0.0, "F0/ORPA"=0.0, "F1/ORPB"=0.0, "F2/ORPK"=0.0, "F3"=0.0, "F4"=0.0, "F5"=0.0, "F6"=0.0, "F7"=0.0, "X0/滴定数"=0.0, "量程"=0.0}, "关键参数改变"=FALSE, "校准信息"={"低标液1浓度"=0.0, "低标液1信号值"=0.0, "低标液1启用"=0, "低标液2浓度"=0.0, "低标液2信号值"=0.0, "低标液2启用"=0, "低标液3浓度"=0.0, "低标液3信号值"=0.0, "低标液3启用"=0, "低标液4浓度"=0.0, "低标液4信号值"=0.0, "低标液4启用"=0, "低标液5浓度"=0.0, "低标液5信号值"=0.0, "低标液5启用"=0, "高标液1浓度"=0.0, "高标液1信号值"=0.0, "高标液1启用"=0, "高标液2浓度"=0.0, "高标液2信号值"=0.0, "高标液2启用"=0, "高标液3浓度"=0.0, "高标液3信号值"=0.0, "高标液3启用"=0, "高标液4浓度"=0.0, "高标液4信号值"=0.0, "高标液4启用"=0, "高标液5浓度"=0.0, "高标液5信号值"=0.0, "高标液5启用"=0, "低斜率"=0.0, "低截距"=0.0, "低二次多项式系数"=0.0, "低线性相关系数"=0.0, "高斜率"=0.0, "高截距"=0.0, "高二次多项式系数"=0.0, "高线性相关系数"=0.0}, "校准信息改变"=FALSE, "固件版本号"=""}  # 与总磷交互全局
      n36 = Obtain Queue(name (unnamed)="总磷 interface Read" ("写入方名称"), element data type=w69) -> (queue out=w70:refnum<queue>)  [unwired: 3 in, 2 out]
    }
  }
  n37 = case shown="真" w9 {
    tunnel: [_ w73] -> w29
    tunnel: [_ w72] -> w28
    frame False {
    }
    frame True {
      w72 = T11 {"状态告警区"={"系统时间"=timestamp(0 s since 1904-01-01), "工作状态"=0, "测量模式"=enum."待机", "告警代码"=0, "故障代码"=0, "日志代码"=0, "软件版本"=0, "F0"=0.0, "F1"=0.0, "F2"=0.0, "F3"=0.0, "T"=0.0, "H"=0.0, "id"=0, "flowid"=0, "量程"=0, "总磷控温温度1"=0.0, "营养盐控温温度2"=0.0, "ADC"=0.0}, "平台试剂余量百分比"=0.0, "关键参数"={"测量量程"=0.0, "测量精度"=0.0, "测量间隔"=0.0, "消解温度"=0.0, "消解时长"=0.0, "空白校准时间"=timestamp(0 s since 1904-01-01), "曲线截距"=0.0, "曲线斜率"=0.0, "测量检出限"=0.0, "测量信号值"=0.0, "线性相关系数"=0.0, "二次多项式系数"=0.0, "标样校准时间"=timestamp(0 s since 1904-01-01), "稀释倍数"=0.0, "三项式系数"=0.0, "空白标定系数"=0.0, "量程系数"=0.0, "F0/ORPA"=0.0, "F1/ORPB"=0.0, "F2/ORPK"=0.0, "F3"=0.0, "F4"=0.0, "F5"=0.0, "F6"=0.0, "F7"=0.0, "X0/滴定数"=0.0, "量程"=0.0}, "关键参数改变"=FALSE, "校准信息"={"低标液1浓度"=0.0, "低标液1信号值"=0.0, "低标液1启用"=0, "低标液2浓度"=0.0, "低标液2信号值"=0.0, "低标液2启用"=0, "低标液3浓度"=0.0, "低标液3信号值"=0.0, "低标液3启用"=0, "低标液4浓度"=0.0, "低标液4信号值"=0.0, "低标液4启用"=0, "低标液5浓度"=0.0, "低标液5信号值"=0.0, "低标液5启用"=0, "高标液1浓度"=0.0, "高标液1信号值"=0.0, "高标液1启用"=0, "高标液2浓度"=0.0, "高标液2信号值"=0.0, "高标液2启用"=0, "高标液3浓度"=0.0, "高标液3信号值"=0.0, "高标液3启用"=0, "高标液4浓度"=0.0, "高标液4信号值"=0.0, "高标液4启用"=0, "高标液5浓度"=0.0, "高标液5信号值"=0.0, "高标液5启用"=0, "低斜率"=0.0, "低截距"=0.0, "低二次多项式系数"=0.0, "低线性相关系数"=0.0, "高斜率"=0.0, "高截距"=0.0, "高二次多项式系数"=0.0, "高线性相关系数"=0.0}, "校准信息改变"=FALSE, "固件版本号"=""}  # 与总氮交互全局
      n38 = Obtain Queue(name (unnamed)="总氮 interface Read" ("写入方名称"), element data type=w72) -> (queue out=w73:refnum<queue>)  [unwired: 3 in, 2 out]
    }
  }
  n39 = case shown="真" w4 {
    tunnel: [_ w76] -> w27
    tunnel: [_ w75] -> w26
    frame False {
    }
    frame True {
      w75 = T12 {"状态告警区"={"系统时间"=timestamp(0 s since 1904-01-01), "工作状态"=0, "测量模式"=enum."待机", "告警代码"=0, "故障代码"=0, "日志代码"=0, "软件版本"=0, "F0"=0.0, "F1"=0.0, "F2"=0.0, "F3"=0.0, "T"=0.0, "H"=0.0, "id"=0, "flowid"=0, "量程"=0, "总磷控温温度1"=0.0, "营养盐控温温度2"=0.0, "ADC"=0.0}, "平台试剂余量百分比"=0.0, "关键参数"={"测量量程"=0.0, "测量精度"=0.0, "测量间隔"=0.0, "消解温度"=0.0, "消解时长"=0.0, "空白校准时间"=timestamp(0 s since 1904-01-01), "曲线截距"=0.0, "曲线斜率"=0.0, "测量检出限"=0.0, "测量信号值"=0.0, "线性相关系数"=0.0, "二次多项式系数"=0.0, "标样校准时间"=timestamp(0 s since 1904-01-01), "稀释倍数"=0.0, "三项式系数"=0.0, "空白标定系数"=0.0, "量程系数"=0.0, "F0/ORPA"=0.0, "F1/ORPB"=0.0, "F2/ORPK"=0.0, "F3"=0.0, "F4"=0.0, "F5"=0.0, "F6"=0.0, "F7"=0.0, "X0/滴定数"=0.0, "量程"=0.0}, "关键参数改变"=FALSE, "校准信息"={"低标液1浓度"=0.0, "低标液1信号值"=0.0, "低标液1启用"=0, "低标液2浓度"=0.0, "低标液2信号值"=0.0, "低标液2启用"=0, "低标液3浓度"=0.0, "低标液3信号值"=0.0, "低标液3启用"=0, "低标液4浓度"=0.0, "低标液4信号值"=0.0, "低标液4启用"=0, "低标液5浓度"=0.0, "低标液5信号值"=0.0, "低标液5启用"=0, "高标液1浓度"=0.0, "高标液1信号值"=0.0, "高标液1启用"=0, "高标液2浓度"=0.0, "高标液2信号值"=0.0, "高标液2启用"=0, "高标液3浓度"=0.0, "高标液3信号值"=0.0, "高标液3启用"=0, "高标液4浓度"=0.0, "高标液4信号值"=0.0, "高标液4启用"=0, "高标液5浓度"=0.0, "高标液5信号值"=0.0, "高标液5启用"=0, "低斜率"=0.0, "低截距"=0.0, "低二次多项式系数"=0.0, "低线性相关系数"=0.0, "高斜率"=0.0, "高截距"=0.0, "高二次多项式系数"=0.0, "高线性相关系数"=0.0}, "校准信息改变"=FALSE, "固件版本号"=""}  # 与氨氮交互全局
      n40 = Obtain Queue(name (unnamed)="氨氮 interface Read" ("写入方名称"), element data type=w75) -> (queue out=w76:refnum<queue>)  [unwired: 3 in, 2 out]
    }
  }
  n41 = Obtain Queue(name (unnamed)=w36, element data type=w41) -> (queue out=w37:refnum<queue>, error out=w40:errorcluster)  [unwired: 3 in, 1 out]
  n42 = while {
    tunnel: w2 -> [w82]
    tunnel: w1 -> [w81]
    tunnel: [w80] -> _
    tunnel: [w79] -> _
    stop <- FALSE stop-if-true
    n43 = for {
      tunnel: w82 -> [w89] mode=indexing
      tunnel: w81 -> [w88] mode=indexing
      tunnel: [w87] -> w80
      tunnel: [w86] -> w79
      n44 = Dequeue Element(queue=w89, timeout in ms (-1)=1000 ("超时毫秒(-1)"), error in (no error)=w88) -> (queue out=w87:refnum<queue>, element=w85:cluster{"selected path":path}, timed out?=w83:bool, error out=w86:errorcluster)
      n45 = case shown="假" w83 {
        tunnel: w85 -> [w98 _]
        frame False {
          n46 = Unbundle By Name(w98) -> ("selected path"=w97:path)
          n47 = call "固件升级（包含参数恢复）.vi"("路径对话框"=FALSE, "selected path"=w97) -> ("结果字符串"=w91:string)  [unwired: 9 in]
          n48 = global read "VAR总磷总氮全局变量.vi" "模块名称"() -> (w93:string)
          n49 = Concatenate Strings("平台反控固件升级" ("日志信息"), w91) -> (w90:string)
          n50 = Get Date/Time In Seconds() -> (seconds since 1Jan1904=w94:timestamp)
          n51 = Bundle By Name(cluster=T13 {"时间"=timestamp(0 s since 1904-01-01), "参数"="", "日志信息"="", "流程参数"=""} ("data in"), "时间"=w94, "参数"=w93, "日志信息"=w90) -> (w95:T13)
          n52 = call "总磷总氮操作日志.vi"("data in"=w95) -> ()  [unwired: 10 in, 1 out]
        }
        frame True {
        }
      }
    }
  }
  n53 = Generate Occurrence() -> (w38:refnum<k4>)
  n54 = while {
    tunnel: w37 -> [w102]
    tunnel: w38 -> [w100]
    stop <- w101 stop-if-true
    n55 = event shown="[5] \"读测量数据区\": 值改变" {
      selector: _ -> [_ _ _ _ _ _ _ _]
      dyn-events: _ -> [_ _ _ _ _ _ _ _]
      timeout: _ -> [_ _ _ _ _ _ _ _]
      tunnel: w102 -> [_ _ _ w133 w140 w146 w151 w156]
      tunnel: [_ _ _ _ "停止" _ _ _] -> w101
      tunnel: w100 -> [_ _ _ _ w137 _ _ _]
      event Timeout {
        n56 = event-data() -> ()  [unwired: 1 in, 3 out]
      }
      event "启用模块": Value Change {
        n57 = event-data() -> ("NewVal"=w103:bool)  [unwired: 1 in, 5 out]
        n58 = call <vilib>:"Application Directory.vi"() -> ("Application Directory"=w105:path)
        n59 = Build Path(base path=w105, name or relative path="data\\set.ini" ("名称或相对路径")) -> (appended path=w106:path)
        n60 = call <vilib>:"Open Config Data.vi"("configuration file path"=w106) -> ("error out"=w112:errorcluster, "refnum"=w111:T14)  [unwired: 8 in, 1 out]
        n61 = call-poly <vilib>:"Write Key.vi"("section"="总磷总氮", "error in (no error)"=w112, "value"=w103, "key"="模块启用", "refnum"=w111) -> ("error out"=w108:errorcluster, "refnum out"=w104:T14)  [unwired: 4 in, 1 out]
        n62 = call <vilib>:"Close Config Data.vi"("error in (no error)"=w108, "refnum"=w104) -> ()  [unwired: 8 in, 2 out]
      }
      event "VISA Resource": Value Change {
        n63 = event-data() -> ()  [unwired: 1 in, 6 out]
        n64 = call <vilib>:"Application Directory.vi"() -> ("Application Directory"=w115:path)
        n65 = Build Path(base path=w115, name or relative path="data\\set.ini" ("名称或相对路径")) -> (appended path=w116:path)
        n66 = call <vilib>:"Open Config Data.vi"("configuration file path"=w116) -> ("error out"=w122:errorcluster, "refnum"=w121:T14)  [unwired: 8 in, 1 out]
        n67 = call-poly <vilib>:"Write Key.vi"("section"="总磷总氮", "error in (no error)"=w122, "value"="VISA Resource", "key"="串口", "refnum"=w121) -> ("error out"=w118:errorcluster, "refnum out"=w114:T14)  [unwired: 4 in, 1 out]
        n68 = call <vilib>:"Close Config Data.vi"("error in (no error)"=w118, "refnum"=w114) -> ()  [unwired: 8 in, 2 out]
      }
      event "启动": Value Change {
        n69 = event-data() -> ()  [unwired: 1 in, 6 out]
        n70 = case shown="默认" "控制命令" {
          tunnel: "控制命令参数" -> [w135 w136]
          tunnel: [w134 w136] -> w123
          frame Default {
            n71 = call "HexToWord.vi"("数组"=w135) -> ("WORD"=w134:u16[])  [unwired: 10 in]
          }
          frame 13 {
          }
        }
        n72 = Swap Bytes(anything="控制命令") -> (byte swapped=w126:u16)
        n73 = call "控制命令区.vi"("控制命令参数"=w123, "控制命令"=w126) -> ("控制命令"=w129:u16[])  [unwired: 9 in]
        n74 = local read "站号"() -> (w128:u16)
        n75 = Bundle("站号"=w128, "控制命令"=w129) -> (w127:cluster{"站号":u16, "控制命令":u16[]})  [unwired: 1 in]
        n76 = Bundle By Name(cluster=cluster{"命令":string, "data":variant} {"命令"="", "data"=variant} ("元素"), "命令"="启动", "data"=w127) -> (w131:cluster{"命令":string, "data":variant})
        n77 = Enqueue Element(queue=w133, element=w131) -> ()  [unwired: 2 in, 3 out]
      }
      event "停止": Value Change {
        n78 = event-data() -> ()  [unwired: 1 in, 6 out]
        n79 = Set Occurrence(w137) -> ()
        n80 = Flush Queue(queue=w140) -> (queue out=w139:refnum<queue>)  [unwired: 1 in, 2 out]
        n81 = Enqueue Element(queue=w139, element=cluster{"命令":string, "data":variant} {"命令"="shutdown", "data"=variant} ("元素")) -> ()  [unwired: 2 in, 3 out]
      }
      event "读测量数据区": Value Change {
        n82 = event-data() -> ()  [unwired: 1 in, 6 out]
        n83 = Bundle By Name(cluster=cluster{"命令":string, "data":variant} {"命令"="", "data"=variant} ("元素"), "命令"="读测量数据区", "data"="站号") -> (w144:cluster{"命令":string, "data":variant})
        n84 = Enqueue Element(queue=w146, element=w144) -> ()  [unwired: 2 in, 3 out]
      }
      event "读状态告警区": Value Change {
        n85 = event-data() -> ()  [unwired: 1 in, 6 out]
        n86 = local read "站号"() -> (w147:u16)
        n87 = Bundle By Name(cluster=cluster{"命令":string, "data":variant} {"命令"="", "data"=variant} ("元素"), "命令"="读状态告警区", "data"=w147) -> (w149:cluster{"命令":string, "data":variant})
        n88 = Enqueue Element(queue=w151, element=w149) -> ()  [unwired: 2 in, 3 out]
      }
      event "读关键参数区": Value Change {
        n89 = event-data() -> ()  [unwired: 1 in, 6 out]
        n90 = local read "站号"() -> (w152:u16)
        n91 = Bundle By Name(cluster=cluster{"命令":string, "data":variant} {"命令"="", "data"=variant} ("元素"), "命令"="读关键参数区", "data"=w152) -> (w154:cluster{"命令":string, "data":variant})
        n92 = Enqueue Element(queue=w156, element=w154) -> ()  [unwired: 2 in, 3 out]
      }
    }
  }
  n93 = while {
    tunnel: w38 -> [w167]
    tunnel: w37 -> [w163]
    stop <- w164 stop-if-true
    n94 = global read "总磷总氮断电保存全局变量.vi" "MB通信方式选择"() -> (w162:enum16{"串口", "TCP"})
    n95 = Wait on Occurrence(2:w167, 3:10000 ("毫秒超时(-1)")) -> (0:w165:bool)  [unwired: 1 in]
    n96 = Not(x=w165) -> (.not. x?=w164:bool)
    n97 = case shown="\"TCP\"" w162 {
      tunnel: [_ w168] -> w159
      frame "串口", Default {
      }
      frame "TCP" {
        n98 = global read "VAR总磷总氮全局变量.vi" "MB session in"() -> (w170:refnum<class "MB_Master.lvclass">)
        n99 = property class="MB_Master"(reference=w170) -> ("Properties:Session Valid"=w169:bool)  [unwired: 1 in, 2 out]
        n100 = Not(x=w169) -> (.not. x?=w168:bool)
      }
    }
    n101 = First Call?() -> (First Call?: T/F=w161:bool)
    n102 = Or(x=w159, y=w161) -> (x .or. y?=w160:bool)
    n103 = local read "启用"() -> (w157:bool)
    n104 = And(x=w157, y=w160) -> (x .and. y?=w158:bool)
    n105 = case shown="真" w158 {
      tunnel: w163 -> [_ w173]
      frame False {
      }
      frame True {
        n106 = Flush Queue(queue=w173) -> (queue out=w171:refnum<queue>)  [unwired: 1 in, 2 out]
        n107 = Enqueue Element(queue=w171, element=cluster{"命令":string, "data":variant} {"命令"="启用模块", "data"=variant} ("元素")) -> ()  [unwired: 2 in, 3 out]
        n108 = property on="VISA Resource" class="VISAName"("DisabledEnum"=T15."Disabled and Grayed Out" ("禁用")) -> ()  [unwired: 2 in, 2 out]
      }
    }
  }
  n109 = while {
    tunnel: w37 -> [w191]
    tunnel: w40 -> [w190]
    shift-right: [w177] -> _
    shift-left: _ -> [w188]
    tunnel: errorcluster {"status"=FALSE, "code"=0, "source"=""} ("error out") -> [w187]
    tunnel: [w183] -> _
    stop <- w189 stop-if-true
    n110 = Dequeue Element(queue=w191, error in (no error)=w190) -> (queue out=w184:refnum<queue>, element=w185:cluster{"命令":string, "data":variant})  [unwired: 1 in, 2 out]
    n111 = Unbundle By Name(w185) -> ("命令"=w186:string, "data"=w181:variant)
    n112 = case shown="\"读状态告警区\"" w186 {
      tunnel: w181 -> [_ _ _ w226 w237 w254 w277 w368 w428 _]
      tunnel: w184 -> [_ _ _ _ _ _ _ _ _ w441]
      tunnel: [_ _ _ _ _ _ _ _ _ TRUE] -> w189
      tunnel: [w194 w197 w213 w229 w240 w256 w281 w376 w435 w437] -> w177
      tunnel: [w195 w196 w214 w228 w239 w255 w282 w367 w436 w438] -> w183
      tunnel: w188 -> [w194 _ w213 w225 w236 w253 w276 w371 w431 w437]
      tunnel: w187 -> [w195 _ w215 w222 w233 w250 w274 w372 w432 w439]
      tunnel: [_ _ _ w217 w230 w244 w266 w349 w422 _] -> w175
      frame Default {
      }
      frame "启用模块" {
        n113 = global read "总磷总氮断电保存全局变量.vi" "MB通信方式选择"() -> (w198:enum16{"串口", "TCP"})
        n114 = case shown="\"TCP\"" w198 {
          tunnel: [w203 w209] -> w196
          tunnel: [w200 w208] -> w197
          frame "串口", Default {
            n115 = global read "总磷总氮断电保存全局变量.vi" "VISA Resource"() -> (w201:refnum<visa-resource-name>)
            n116 = call <vilib>:"Open Serial Session.vi"("Mode (RTU)"=enum16{"RTU", "ASCII"}."RTU", "Slave ID"=u8 1, "Serial Config"=T16 {"baud rate (bps)"=115200, "stop bits"=10, "parity"=0, "flow control"=0, "timeout"=1000, "retries"=1}, "VISA Resource"=w201) -> ("Error out"=w203:errorcluster, "MB_Serial session"=w200:refnum<class "MB_Master_Serial.lvclass">)  [unwired: 6 in]
          }
          frame "TCP" {
            n117 = global read "总磷总氮断电保存全局变量.vi" "PORT"() -> (w207:string)
            n118 = Decimal String To Number(string=w207) -> (number=w210:i32)  [unwired: 2 in, 1 out]
            n119 = global read "总磷总氮断电保存全局变量.vi" "IP"() -> (w206:string)
            n120 = call <vilib>:"Open TCP Session.vi"("Port (502)"=w210, "IP Address"=w206) -> ("error out"=w209:errorcluster, "MB_TCP session"=w208:refnum<class "MB_Master_TCP.lvclass">)  [unwired: 8 in]
          }
        }
        "启用" <- TRUE
      }
      frame "停用模块" {
        n121 = call-dynamic "Close Session.vi"("error in (no error)"=w215, "MB session in"=w213) -> ("error out"=w211:errorcluster)  [unwired: 9 in]
        n122 = local write "启用"(FALSE ("启用")) -> ()
        n123 = call <vilib>:"Clear Errors.vi"("error in (no error)"=w211) -> ("error out"=w214:errorcluster)  [unwired: 5 in, 1 out]
      }
      frame "启动" {
        n124 = Variant To Data(type=cluster{"站号":u16, "控制命令":u16[]} {"站号"=0, "控制命令"=[]} ("输出簇"), Variant=w226) -> (data=w220:cluster{"站号":u16, "控制命令":u16[]})  [unwired: 1 in, 1 out]
        n125 = Unbundle By Name(w220) -> ("站号"=w217:u16, "控制命令"=w218:u16[])
        n126 = property class="MB_Master"(reference=w225, error in=w222, "Properties:Slave ID"=w217) -> (reference out=w224:refnum<class "MB_Master.lvclass">, error out=w223:errorcluster)
        n127 = Index Array(array=w218) -> (element=w219:u16)  [unwired: 1 in]
        n128 = Swap Bytes(anything=w219) -> (byte swapped=w216:u16)
        n129 = global write "VAR总磷总氮全局变量.vi" "控制命令"(w216) -> ()
        n130 = call <vilib>:"Write Multiple Registers.vi"("error in (no error)"=w223, "values"=w218, "starting address"=u16 4608, "MB session in"=w224) -> ("error out"=w228:errorcluster, "MB session out"=w229:refnum<class "MB_Master.lvclass">)  [unwired: 6 in]
      }
      frame "盲样测试" {
        n131 = Variant To Data(type=u8 0, Variant=w237) -> (data=w230:u8)  [unwired: 1 in, 1 out]
        n132 = property class="MB_Master"(reference=w236, error in=w233, "Properties:Slave ID"=w230) -> (reference out=w235:refnum<class "MB_Master.lvclass">, error out=w234:errorcluster)
        n133 = case shown="默认" w230 {
          tunnel: [u16[] [] ("values") u16[] [33539, 0] ("values") u16[] [23555, 0] ("values")] -> w232
          frame Default {
          }
          frame 1 {
            # "总磷盲样测试命令"
          }
          frame 3 {
            # "氨氮盲样测试"
          }
        }
        n134 = call <vilib>:"Write Multiple Registers.vi"("error in (no error)"=w234, "values"=w232, "starting address"=u16 24592, "MB session in"=w235) -> ("error out"=w239:errorcluster, "MB session out"=w240:refnum<class "MB_Master.lvclass">)  [unwired: 6 in]
      }
      frame "debug" {
        n135 = Variant To Data(type=cluster{"站号":u16, "控制命令":u16[]} {"站号"=0, "控制命令"=[]} ("输出簇"), Variant=w254) -> (data=w248:cluster{"站号":u16, "控制命令":u16[]})  [unwired: 1 in, 1 out]
        n136 = Unbundle By Name(w248) -> ("站号"=w244:u16, "控制命令"=w246:u16[])
        n137 = property class="MB_Master"(reference=w253, error in=w250, "Properties:Slave ID"=w244) -> (reference out=w252:refnum<class "MB_Master.lvclass">, error out=w251:errorcluster)
        n138 = Index Array(array=w246) -> (element=w247:u16)  [unwired: 1 in]
        n139 = global write "VAR总磷总氮全局变量.vi" "控制命令"(w247) -> ()
        n140 = call <vilib>:"Write Multiple Registers.vi"("error in (no error)"=w251, "values"=w246, "starting address"=u16 24594, "MB session in"=w252) -> ("error out"=w255:errorcluster, "MB session out"=w256:refnum<class "MB_Master.lvclass">)  [unwired: 6 in]
      }
      frame "读测量数据区" {
        n141 = Variant To Data(type=u8 1 ("Slave ID"), Variant=w277) -> (data=w266:u8)  [unwired: 1 in, 1 out]
        n142 = property class="MB_Master"(reference=w276, error in=w274, "Properties:Slave ID"=w266) -> (reference out=w275:refnum<class "MB_Master.lvclass">, error out=w273:errorcluster)
        n143 = global read "VAR总磷总氮全局变量.vi" "测量数据区数组"() -> (w270:T8)
        n144 = call "id参数转换.vi"("id"=w266) -> ("数组资源索引"=w265:i32)  [unwired: 9 in, 1 out]
        n145 = call <vilib>:"Read Holding Registers.vi"("error in (no error)"=w273, "quantity"=u16 107, "starting address"=u16 4096, "MB session in"=w275) -> ("error out"=w282:errorcluster, "Registers"=w272:u16[], "MB session out"=w281:refnum<class "MB_Master.lvclass">)  [unwired: 5 in]
        n146 = call "id参数转换.vi"("id"=u16 2) -> ("数组资源索引"=w262:i32)  [unwired: 9 in, 1 out]
        n147 = call "id参数转换.vi"("id"=u16 3) -> ("数组资源索引"=w260:i32)  [unwired: 9 in, 1 out]
        n148 = Index Array(array=w270, index #1=w265, index #2=w262, index #3=w260) -> (element #1=w271:T5, element #2=w267:T5, element #3=w264:T5)
        n149 = call "测量数据区.vi"("数组"=w272) -> ("测量数据区"=w257:T5)  [unwired: 10 in]
        "测量数据区" <- w257
        n150 = global write "VAR总磷总氮全局变量.vi" "测量数据区"(w257) -> ()
        n151 = global read "工况数据接口全局.vi" "data"() -> (w259:T17)
        n152 = case shown="22" w266 {
          tunnel: w257 -> [w284 w291 w332 w340 w347]
          tunnel: w272 -> [_ w304 w333 w341 w348]
          tunnel: w271 -> [_ w297 _ _ _]
          tunnel: [w284 w299 w332 w340 w347] -> w269
          tunnel: w267 -> [_ w295 _ _ _]
          tunnel: w264 -> [_ w294 _ _ _]
          tunnel: w259 -> [w283 w292 w331 w339 w346]
          tunnel: [w283 w285 w320 w334 w345] -> w258
          tunnel: w257 -> [_ _ w330 w338 w344]
          frame 0, Default {
          }
          frame 1 {
            n153 = Unbundle By Name(w291) -> ("F0"=w290:sgl, "F1"=w289:sgl, "F2"=w288:sgl, "F3"=w287:sgl, "X值"=w286:sgl)
            n154 = Bundle By Name(cluster=w292, "data.TP.TP.F0"=w290, "data.TP.TP.F1"=w289, "data.TP.TP.F2"=w288, "data.TP.TP.F3"=w287, "data.TP.TP.X0"=w286) -> (w285:T17)
            n155 = global read "VAR总磷总氮全局变量.vi" "模块名称"() -> (w303:string)
            n156 = Search and Replace String(input string=w303, search string="总磷" ("搜索字符串")) -> (result string=w300:string, offset past replacement=w301:i32)  [unwired: 6 in, 2 out]
            n157 = case shown="默认" w301 {
              tunnel: w300 -> [_ w310]
              tunnel: [_ w307] -> w298
              tunnel: [_ w305] -> w296
              frame -1 {
              }
              frame Default {
                n158 = Search and Replace String(input string=w310, search string="总氮" ("搜索字符串")) -> (offset past replacement=w313:i32)  [unwired: 6 in, 3 out]
                n159 = Search and Replace String(input string=w310, search string="氨氮" ("搜索字符串")) -> (offset past replacement=w308:i32)  [unwired: 6 in, 3 out]
                n160 = Not Equal?(x=w313, y=-1) -> (x != y?=w305:bool)
                n161 = Not Equal?(x=w308, y=-1) -> (x != y?=w306:bool)
                n162 = Or(x=w306, y=w305) -> (x .or. y?=w307:bool)
              }
            }
            n163 = Select(t=w295, s=w296, f=w294) -> (s? t:f=w293:T5)
            n164 = case shown="真" w298 {
              tunnel: [w315 w319] -> w299
              tunnel: w297 -> [_ w318]
              tunnel: w293 -> [_ w317]
              tunnel: w291 -> [w315 w316]
              frame False {
              }
              frame True {
                # "启动总磷总氮时间自动对齐"
                n165 = call "数据时间对齐.vi"("待对齐时间"=w316, "对齐参考时间"=w317, "已对齐时间输入"=w318) -> ("已对齐时间输出"=w319:T5)  [unwired: 8 in]
              }
            }
            "总磷测量数据区" <- w304
          }
          frame 2 {
            n166 = Unbundle By Name(w330) -> ("F0"=w329:sgl, "F1"=w328:sgl, "F2"=w327:sgl, "F3"=w326:sgl, "F4"=w325:sgl, "F5"=w324:sgl, "F6"=w323:sgl, "F7"=w322:sgl, "X值"=w321:sgl)
            n167 = Bundle By Name(cluster=w331, "data.TN.TN.F0"=w329, "data.TN.TN.F1"=w328, "data.TN.TN.F2"=w327, "data.TN.TN.F3"=w326, "data.TN.TN.F4"=w325, "data.TN.TN.F5"=w324, "data.TN.TN.F6"=w323, "data.TN.TN.F7"=w322, "data.TN.TN.X0"=w321) -> (w320:T17)
            "总氮测量数据区" <- w333
          }
          frame 3 {
            n168 = Unbundle By Name(w338) -> ("F0"=w337:sgl, "F1"=w336:sgl, "X值"=w335:sgl)
            n169 = Bundle By Name(cluster=w339, "data.NH3.NH3.F0"=w337, "data.NH3.NH3.F1"=w336, "data.NH3.NH3.X0"=w335) -> (w334:T17)
            "氨氮测量数据区" <- w341
          }
          frame 22 {
            n170 = Unbundle By Name(w344) -> ("F0"=w343:sgl, "F1"=w342:sgl)
            n171 = Bundle By Name(cluster=w346, "data.CODCr.CODCr.F0"=w343, "data.CODCr.CODCr.F1"=w342) -> (w345:T17)
            "COD测量数据区" <- w348
          }
        }
        n172 = global write "工况数据接口全局.vi" "data"(w258) -> ()
        n173 = Replace Array Subset(array=w270, new element=w269, index=w265) -> (w268:T8)
        n174 = global write "VAR总磷总氮全局变量.vi" "测量数据区数组"(w268) -> ()
      }
      frame "读状态告警区" {
        n175 = Variant To Data(type=u8 1 ("Slave ID"), Variant=w368) -> (data=w349:u8)  [unwired: 1 in, 1 out]
        n176 = property class="MB_Master"(reference=w371, error in=w372, "Properties:Slave ID"=w349) -> (reference out=w370:refnum<class "MB_Master.lvclass">, error out=w369:errorcluster)
        n177 = call "id参数转换.vi"("id"=w349) -> ("数组资源索引"=w362:i32)  [unwired: 9 in, 1 out]
        n178 = call <vilib>:"Read Holding Registers.vi"("error in (no error)"=w369, "quantity"=u16 44, "starting address"=u16 4224, "MB session in"=w370) -> ("error out"=w367:errorcluster, "Registers"=w365:u16[], "MB session out"=w376:refnum<class "MB_Master.lvclass">)  [unwired: 5 in]
        n179 = global read "VAR总磷总氮全局变量.vi" "状态告警区数组"() -> (w364:T7)
        n180 = call "状态告警区.vi"("数组"=w365) -> ("状态告警区 2"=w350:T18, "状态告警区"=w351:T4)  [unwired: 9 in]
        "状态告警区" <- w350
        n181 = Unbundle By Name(w351) -> ("日志代码"=w352:u16, "告警代码"=w358:u16, "故障代码"=w356:u16)
        n182 = global write "VAR总磷总氮全局变量.vi" "状态告警区"(w350) -> ()
        n183 = Unbundle By Name(w351) -> ("id"=w366:u16)
        n184 = Replace Array Subset(array=w364, new element=w351, index=w362) -> (w363:T7)
        n185 = global write "VAR总磷总氮全局变量.vi" "状态告警区数组"(w363) -> ()
        n186 = feedback-in #1(w358) -> ()
        n187 = feedback #1() -> (w359:u16)  [unwired: 1 in]
        n188 = feedback #2() -> (w357:u16)  [unwired: 1 in]
        n189 = feedback-in #2(w356) -> ()
        n190 = Not Equal?(x=w359, y=w358) -> (x != y?=w355:bool)
        n191 = Not Equal?(x=w357, y=w356) -> (x != y?=w354:bool)
        n192 = Or(x=w355, y=w354) -> (x .or. y?=w353:bool)
        n193 = global read "工况数据接口全局.vi" "data"() -> (w361:T17)
        n194 = case shown="2, 76" w366 {
          tunnel: w351 -> [_ w389 w402 w412 w418]
          tunnel: w365 -> [_ w390 w403 w413 w420]
          tunnel: w361 -> [w377 w380 w395 w408 w419]
          tunnel: [w377 w387 w397 w411 w416] -> w360
          tunnel: w353 -> [_ w382 w393 w407 _]
          tunnel: w352 -> [_ w381 w392 w406 _]
          frame 0, Default {
          }
          frame 1, 131 {
            n195 = Unbundle By Name(w380) -> ("data.TP.TP.alarm_step"=w379:dbl)
            n196 = Unbundle By Name(w389) -> ("总磷控温温度1"=w388:sgl, "营养盐控温温度2"=w384:sgl)
            n197 = Select(t=w381, s=w382, f=w379) -> (s? t:f=w378:dbl)
            n198 = global read "VAR总磷总氮全局变量.vi" "总磷关键参数"() -> (w386:T19)
            n199 = Unbundle By Name(w386) -> ("消解温度"=w385:sgl)
            n200 = Bundle By Name(cluster=w380, "data.TP.TP.alarm_step"=w378, "data.TP.TP.digestion_temperature"=w388, "data.TP.TP.constant_temperature"=w385, "data.TP.TP.syringe_temperature"=w384, "data.TP.启用"=TRUE) -> (w387:T17)
            "总磷状态告警区" <- w390
          }
          frame 2, 76 {
            n201 = Unbundle By Name(w395) -> ("data.TN.TN.alarm_step"=w394:dbl)
            n202 = Unbundle By Name(w402) -> ("总磷控温温度1"=w398:sgl, "营养盐控温温度2"=w400:sgl)
            n203 = Select(t=w392, s=w393, f=w394) -> (s? t:f=w391:dbl)
            n204 = global read "VAR总磷总氮全局变量.vi" "总氮关键参数"() -> (w401:T19)
            n205 = Unbundle By Name(w401) -> ("消解温度"=w399:sgl)
            n206 = Bundle By Name(cluster=w395, "data.TN.TN.alarm_step"=w391, "data.TN.TN.digestion_temperature"=w398, "data.TN.TN.constant_temperature"=w399, "data.TN.TN.syringe_temperature"=w400, "data.TN.启用"=TRUE) -> (w397:T17)
            "总氮状态告警区" <- w403
          }
          frame 3 {
            n207 = Unbundle By Name(w408) -> ("data.NH3.NH3.alarm_step"=w405:dbl)
            n208 = Unbundle By Name(w412) -> ("营养盐控温温度2"=w410:sgl)
            n209 = Select(t=w406, s=w407, f=w405) -> (s? t:f=w404:dbl)
            n210 = Bundle By Name(cluster=w408, "data.NH3.NH3.alarm_step"=w404, "data.NH3.NH3.syringe_temperature"=w410, "data.NH3.启用"=TRUE) -> (w411:T17)
            "氨氮状态告警区" <- w413
          }
          frame 22 {
            n211 = Unbundle By Name(w418) -> ("营养盐控温温度2"=w417:sgl)
            n212 = global read "VAR总磷总氮全局变量.vi" "波形图-消解温度"() -> (w414:sgl[])
            n213 = Bundle By Name(cluster=w419, "data.CODCr.CODCr.temperature_curve"=w414, "data.CODCr.CODCr.reagent_sensor"=w417, "data.CODCr.启用"=TRUE) -> (w416:T17)
            "COD状态告警区" <- w420
          }
        }
        n214 = global write "工况数据接口全局.vi" "data"(w360) -> ()
      }
      frame "读关键参数区" {
        n215 = Variant To Data(type=u8 1 ("Slave ID"), Variant=w428) -> (data=w422:u8)  [unwired: 1 in, 1 out]
        n216 = property class="MB_Master"(reference=w431, error in=w432, "Properties:Slave ID"=w422) -> (reference out=w430:refnum<class "MB_Master.lvclass">, error out=w429:errorcluster)
        n217 = call "id参数转换.vi"("id"=w422) -> ("数组资源索引"=w421:i32)  [unwired: 9 in, 1 out]
        n218 = call <vilib>:"Read Holding Registers.vi"("error in (no error)"=w429, "quantity"=u16 19, "starting address"=u16 4256, "MB session in"=w430) -> ("error out"=w436:errorcluster, "Registers"=w426:u16[], "MB session out"=w435:refnum<class "MB_Master.lvclass">)  [unwired: 5 in]
        n219 = global read "VAR总磷总氮全局变量.vi" "关键参数区数组"() -> (w425:T6)
        n220 = call "关键参数区.vi"("数组"=w426) -> ("关键参数区"=w424:T3)  [unwired: 10 in]
        "关键参数区" <- w424
        n221 = global write "VAR总磷总氮全局变量.vi" "关键参数区"(w424) -> ()
        n222 = Replace Array Subset(array=w425, new element=w424, index=w421) -> (w423:T6)
        n223 = global write "VAR总磷总氮全局变量.vi" "关键参数区数组"(w423) -> ()
      }
      frame "shutdown" {
        n224 = call-dynamic "Close Session.vi"("error in (no error)"=w439, "MB session in"=w437) -> ("error out"=w438:errorcluster)  [unwired: 9 in]
        n225 = Flush Queue(queue=w441) -> (queue out=w440:refnum<queue>)  [unwired: 1 in, 2 out]
        n226 = Release Queue(queue=w440) -> ()  [unwired: 2 in, 3 out]
      }
    }
    n227 = global write "VAR总磷总氮全局变量.vi" "MB session in"(w177) -> ()
    n228 = Unbundle By Name(w183) -> ("status"=w180:bool)
    n229 = Not(x=w180) -> (.not. x?=w182:bool)
    "status" <- w182
    n230 = call <vilib>:"Boolean Crossing PtByPt.vi"("direction"=enum16{"either", "false-true", "true-false"}."false-true", "input"=w180) -> ("crossing"=w179:bool)  [unwired: 1 in]
    n231 = case shown="假" w179 {
      tunnel: [u16 0 ("告警代码") u16 999 ("告警代码")] -> w176
      frame False {
      }
      frame True {
      }
    }
    n232 = global write "VAR总磷总氮全局变量.vi" "通讯状态"(w182) -> ()
    n233 = call "告警码字段定义.vi"("id"=w175, "告警代码"=w176) -> ()  [unwired: 9 in, 1 out]
  }
  n234 = while {
    tunnel: w35 -> [w453]
    tunnel: w34 -> [w452]
    tunnel: w33 -> [w451]
    tunnel: w32 -> [w450]
    tunnel: w31 -> [w449]
    tunnel: w30 -> [w448]
    tunnel: w29 -> [w447]
    tunnel: w28 -> [w446]
    tunnel: w27 -> [w445]
    tunnel: w26 -> [w444]
    stop <- FALSE stop-if-true
    n235 = global read "model config var.vi" "启动队列名称"() -> (w456:cluster{"String":string, "Value":u16}[])
    n236 = Wait (ms)(milliseconds to wait=u32 1000 ("等待时间（毫秒）")) -> ()  [unwired: 1 out]
    n237 = global read "VAR总磷总氮全局变量.vi" "固件版本号"() -> (w443:string)
    n238 = for {
      tunnel: w456 -> [w469] mode=indexing
      tunnel: w453 -> [w467]
      tunnel: w452 -> [w466]
      tunnel: w451 -> [w465]
      tunnel: w450 -> [w464]
      tunnel: w449 -> [w463]
      tunnel: w448 -> [w462]
      tunnel: w447 -> [w461]
      tunnel: w446 -> [w460]
      tunnel: w445 -> [w459]
      tunnel: w444 -> [w458]
      tunnel: w443 -> [w457]
      n239 = Unbundle By Name(w469) -> ("Value"=w468:u16)
      n240 = case shown="1" w468 {
        tunnel: w467 -> [_ _ _ _ w556 _]
        tunnel: w466 -> [_ _ _ _ w555 _]
        tunnel: w465 -> [_ _ _ w535 _ _]
        tunnel: w464 -> [_ _ _ w534 _ _]
        tunnel: w463 -> [w472 _ _ _ _ _]
        tunnel: w462 -> [w471 _ _ _ _ _]
        tunnel: w461 -> [_ w493 _ _ _ _]
        tunnel: w460 -> [_ w492 _ _ _ _]
        tunnel: w459 -> [_ _ w514 _ _ _]
        tunnel: w458 -> [_ _ w513 _ _ _]
        tunnel: w457 -> [w470 w491 w512 w533 w554 _]
        frame 1 {
          n241 = Get Queue Status(queue=w472) -> (queue out=w475:refnum<queue>, # elements in queue=w474:i32)  [unwired: 2 in, 6 out]
          n242 = Equal To 0?(x=w474) -> (x = 0?=w473:bool)
          n243 = case shown="真" w473 {
            tunnel: w471 -> [_ w487]
            tunnel: w475 -> [_ w488]
            tunnel: w470 -> [_ w476]
            frame False {
            }
            frame True {
              w478 = u16 1 items=["总磷"=1, "总氮"=2, "氨氮"=3, "磷酸盐"=4, "硝氮"=5, "亚硝氮"=6, "硅酸盐"=7, "硫化物"=8, "CODCr"=22]
              n244 = Unbundle By Name(w487) -> ("关键参数"=w485:T20)
              n245 = global read "VAR总磷总氮全局变量.vi" "总磷关键参数"() -> (w486:T19)
              n246 = global read "VAR总磷总氮全局变量.vi" "状态告警区数组"() -> (w480:T7)
              n247 = global read "VAR总磷总氮全局变量.vi" "平台试剂余量百分比"() -> (w490:sgl)
              n248 = call "id参数转换.vi"("id"=w478) -> ("数组资源索引"=w479:i32)  [unwired: 9 in, 1 out]
              n249 = call "转换关键参数(子VI).vi"("参数"=w478, "总磷关键参数"=w486, "关键参数输入"=w485) -> ("关键参数输出"=w484:T20)  [unwired: 8 in]
              n250 = global read "VAR总磷总氮全局变量.vi" "总磷关键参数改变"() -> (w483:bool)
              n251 = global read "VAR总磷总氮全局变量.vi" "总磷校准信息改变"() -> (w481:bool)
              n252 = global read "VAR总磷总氮全局变量.vi" "总磷校准信息"() -> (w482:T21)
              n253 = Index Array(array=w480, index=w479) -> (element=w477:T4)
              n254 = Bundle By Name(cluster=w487, "状态告警区"=w477, "平台试剂余量百分比"=w490, "关键参数"=w484, "关键参数改变"=w483, "校准信息"=w482, "校准信息改变"=w481, "固件版本号"=w476) -> (w489:T10)
              n255 = Enqueue Element(queue=w488, element=w489) -> ()  [unwired: 2 in, 3 out]
            }
          }
        }
        frame 2 {
          n256 = Get Queue Status(queue=w493) -> (queue out=w496:refnum<queue>, # elements in queue=w495:i32)  [unwired: 2 in, 6 out]
          n257 = Equal To 0?(x=w495) -> (x = 0?=w494:bool)
          n258 = case shown="真" w494 {
            tunnel: w496 -> [_ w509]
            tunnel: w492 -> [_ w507]
            tunnel: w491 -> [_ w497]
            frame False {
            }
            frame True {
              w499 = u16 2 items=["总磷"=1, "总氮"=2, "氨氮"=3, "磷酸盐"=4, "硝氮"=5, "亚硝氮"=6, "硅酸盐"=7, "硫化物"=8, "CODCr"=22]
              n259 = Unbundle By Name(w507) -> ("关键参数"=w506:T20)
              n260 = global read "VAR总磷总氮全局变量.vi" "总氮关键参数"() -> (w508:T19)
              n261 = global read "VAR总磷总氮全局变量.vi" "状态告警区数组"() -> (w500:T7)
              n262 = global read "VAR总磷总氮全局变量.vi" "平台试剂余量百分比"() -> (w511:sgl)
              n263 = call "id参数转换.vi"("id"=w499) -> ("数组资源索引"=w501:i32)  [unwired: 9 in, 1 out]
              n264 = call "转换关键参数(子VI).vi"("参数"=w499, "总磷关键参数"=w508, "关键参数输入"=w506) -> ("关键参数输出"=w505:T20)  [unwired: 8 in]
              n265 = global read "VAR总磷总氮全局变量.vi" "总氮关键参数改变"() -> (w504:bool)
              n266 = global read "VAR总磷总氮全局变量.vi" "总氮校准信息改变"() -> (w502:bool)
              n267 = global read "VAR总磷总氮全局变量.vi" "总氮校准信息"() -> (w503:T21)
              n268 = Index Array(array=w500, index=w501) -> (element=w498:T4)
              n269 = Bundle By Name(cluster=w507, "状态告警区"=w498, "平台试剂余量百分比"=w511, "关键参数"=w505, "关键参数改变"=w504, "校准信息"=w503, "校准信息改变"=w502, "固件版本号"=w497) -> (w510:T11)
              n270 = Enqueue Element(queue=w509, element=w510) -> ()  [unwired: 2 in, 3 out]
            }
          }
        }
        frame 3 {
          (unwired) FALSE
          n271 = Get Queue Status(queue=w514) -> (queue out=w516:refnum<queue>, # elements in queue=w517:i32)  [unwired: 2 in, 6 out]
          n272 = Equal To 0?(x=w517) -> (x = 0?=w515:bool)
          n273 = case shown="真" w515 {
            tunnel: w516 -> [_ w530]
            tunnel: w513 -> [_ w529]
            tunnel: w512 -> [_ w518]
            frame False {
            }
            frame True {
              w520 = u16 3 items=["总磷"=1, "总氮"=2, "氨氮"=3, "磷酸盐"=4, "硝氮"=5, "亚硝氮"=6, "硅酸盐"=7, "硫化物"=8, "CODCr"=22]
              n274 = Unbundle By Name(w529) -> ("关键参数"=w528:T20)
              n275 = global read "VAR总磷总氮全局变量.vi" "氨氮关键参数"() -> (w526:T19)
              n276 = global read "VAR总磷总氮全局变量.vi" "状态告警区数组"() -> (w521:T7)
              n277 = global read "VAR总磷总氮全局变量.vi" "平台试剂余量百分比"() -> (w532:sgl)
              n278 = call "id参数转换.vi"("id"=w520) -> ("数组资源索引"=w522:i32)  [unwired: 9 in, 1 out]
              n279 = call "转换关键参数(子VI).vi"("参数"=w520, "总磷关键参数"=w526, "关键参数输入"=w528) -> ("关键参数输出"=w527:T20)  [unwired: 8 in]
              n280 = global read "VAR总磷总氮全局变量.vi" "氨氮关键参数改变"() -> (w525:bool)
              n281 = global read "VAR总磷总氮全局变量.vi" "氨氮校准信息改变"() -> (w523:bool)
              n282 = global read "VAR总磷总氮全局变量.vi" "氨氮校准信息"() -> (w524:T21)
              n283 = Index Array(array=w521, index=w522) -> (element=w519:T4)
              n284 = Bundle By Name(cluster=w529, "状态告警区"=w519, "平台试剂余量百分比"=w532, "关键参数"=w527, "关键参数改变"=w525, "校准信息"=w524, "校准信息改变"=w523, "固件版本号"=w518) -> (w531:T12)
              n285 = Enqueue Element(queue=w530, element=w531) -> ()  [unwired: 2 in, 3 out]
            }
          }
        }
        frame 22 {
          n286 = Get Queue Status(queue=w535) -> (queue out=w537:refnum<queue>, # elements in queue=w538:i32)  [unwired: 2 in, 6 out]
          n287 = Equal To 0?(x=w538) -> (x = 0?=w536:bool)
          n288 = case shown="真" w536 {
            tunnel: w537 -> [_ w551]
            tunnel: w534 -> [_ w550]
            tunnel: w533 -> [_ w539]
            frame False {
            }
            frame True {
              w541 = u16 22 items=["总磷"=1, "总氮"=2, "氨氮"=3, "磷酸盐"=4, "硝氮"=5, "亚硝氮"=6, "硅酸盐"=7, "硫化物"=8, "CODCr"=22]
              n289 = Unbundle By Name(w550) -> ("关键参数"=w549:T20)
              n290 = global read "VAR总磷总氮全局变量.vi" "CODcr关键参数"() -> (w548:T19)
              n291 = global read "VAR总磷总氮全局变量.vi" "状态告警区数组"() -> (w542:T7)
              n292 = global read "VAR总磷总氮全局变量.vi" "CODCr关键参数改变"() -> (w546:bool)
              n293 = global read "VAR总磷总氮全局变量.vi" "CODCr校准信息改变"() -> (w544:bool)
              n294 = global read "VAR总磷总氮全局变量.vi" "平台试剂余量百分比"() -> (w553:sgl)
              n295 = call "id参数转换.vi"("id"=w541) -> ("数组资源索引"=w543:i32)  [unwired: 9 in, 1 out]
              n296 = call "转换关键参数(子VI).vi"("参数"=w541, "总磷关键参数"=w548, "关键参数输入"=w549) -> ("关键参数输出"=w547:T20)  [unwired: 8 in]
              n297 = global read "VAR总磷总氮全局变量.vi" "CODCr校准信息"() -> (w545:T21)
              n298 = Index Array(array=w542, index=w543) -> (element=w540:T4)
              n299 = Bundle By Name(cluster=w550, "状态告警区"=w540, "平台试剂余量百分比"=w553, "关键参数"=w547, "关键参数改变"=w546, "校准信息"=w545, "校准信息改变"=w544, "固件版本号"=w539) -> (w552:T9)
              n300 = Enqueue Element(queue=w551, element=w552) -> ()  [unwired: 2 in, 3 out]
            }
          }
        }
        frame 21 {
          (unwired) FALSE
          n301 = Get Queue Status(queue=w556) -> (queue out=w558:refnum<queue>, # elements in queue=w559:i32)  [unwired: 2 in, 6 out]
          n302 = Equal To 0?(x=w559) -> (x = 0?=w557:bool)
          n303 = case shown="真" w557 {
            tunnel: w558 -> [_ w572]
            tunnel: w555 -> [_ w571]
            tunnel: w554 -> [_ w560]
            frame False {
            }
            frame True {
              w562 = u16 21 items=["总磷"=1, "总氮"=2, "氨氮"=3, "磷酸盐"=4, "硝氮"=5, "亚硝氮"=6, "硅酸盐"=7, "硫化物"=8, "CODMn"=21, "CODCr"=22, "氟化物"=50]
              n304 = Unbundle By Name(w571) -> ("关键参数"=w570:T20)
              n305 = global read "VAR总磷总氮全局变量.vi" "CODMn关键参数"() -> (w569:T19)
              n306 = global read "VAR总磷总氮全局变量.vi" "状态告警区数组"() -> (w563:T7)
              n307 = global read "VAR总磷总氮全局变量.vi" "CODmn关键参数改变"() -> (w567:bool)
              n308 = global read "VAR总磷总氮全局变量.vi" "CODMn校准信息改变"() -> (w565:bool)
              n309 = global read "VAR总磷总氮全局变量.vi" "平台试剂余量百分比"() -> (w574:sgl)
              n310 = call "id参数转换.vi"("id"=w562) -> ("数组资源索引"=w564:i32)  [unwired: 9 in, 1 out]
              n311 = call "转换关键参数(子VI).vi"("参数"=w562, "总磷关键参数"=w569, "关键参数输入"=w570) -> ("关键参数输出"=w568:T20)  [unwired: 8 in]
              n312 = global read "VAR总磷总氮全局变量.vi" "CODMn校准信息"() -> (w566:T21)
              n313 = Index Array(array=w563, index=w564) -> (element=w561:T4)
              n314 = Bundle By Name(cluster=w571, "状态告警区"=w561, "平台试剂余量百分比"=w574, "关键参数"=w568, "关键参数改变"=w567, "校准信息"=w566, "校准信息改变"=w565, "固件版本号"=w560) -> (w573:T9)
              n315 = Enqueue Element(queue=w572, element=w573) -> ()  [unwired: 2 in, 3 out]
            }
          }
        }
        frame Default {
        }
      }
    }
  }
